vi "EnFlo_Hub.vi"() -> ()   [LabVIEW 2022 SP3]
uses:
  Anemometry Sub Vis/Controls/Launch_controls/Open_Calib.ctl
  Anemometry Sub Vis/Controls/Launch_controls/Open_Meas.ctl
  Anemometry Sub Vis/Controls/Launch_controls/Open_Enter_Temp.ctl
  Anemometry Sub Vis/Controls/Launch_controls/Multi_Run_Prog.ctl
  Anemometry Sub Vis/Controls/Launch_controls/EnFlo_arm.ctl
  Anemometry Sub Vis/Controls/Launch_controls/Disp_Setup.ctl
  Anemometry Sub Vis/Controls/Launch_controls/EnFlo_Tun_Setup.ctl
  Anemometry Sub Vis/Controls/Launch_controls/User_Metadata.ctl
  Anemometry Sub Vis/Controls/Launch_controls/Trav_3D_move.ctl
  Anemometry Sub Vis/Controls/Launch_controls/Trav_Space.ctl
  Anemometry Sub Vis/Controls/Launch_controls/Tunnel_speed.ctl
  Anemometry Sub Vis/Controls/Launch_controls/Client_source_control.ctl
  Anemometry Sub Vis/Controls/Launch_controls/Hydrosonic_Manual.ctl
  Anemometry Sub Vis/Controls/Launch_controls/Preference_Panel.ctl
  Anemometry Sub Vis/Controls/Launch_controls/Hot_wire_Calculator.ctl
  Anemometry Sub Vis/Controls/Launch_controls/RW_X_Parker_Config.ctl
  Anemometry Sub Vis/Controls/Launch_controls/LDA_Alignment.ctl
  Anemometry Sub Vis/Controls/Launch_controls/Named_Serial_Comms.ctl
  Anemometry Sub Vis/Controls/Launch_controls/BSA_data_rates.ctl
  Anemometry Sub Vis/Controls/Launch_controls/Serial_Setup.ctl
  Anemometry Sub Vis/Controls/Launch_controls/Post_Process_icon.ctl
  Anemometry Sub Vis/Controls/Launch_controls/Edit_Ascii_file.ctl
  Anemometry Sub Vis/Controls/Launch_controls/Edit_Raw_DF.ctl
  Anemometry Sub Vis/Controls/Launch_controls/Results_file_plotter.ctl
  Anemometry Sub Vis/Controls/Launch_controls/Serial_Port_Names.ctl
  Anemometry Sub Vis/Controls/Launch_controls/Paul.ctl
  Anemometry Sub Vis/Controls/Launch_controls/Tom.ctl
  Anemometry Sub Vis/Controls/Launch_controls/Scani_Valve.ctl
  Anemometry Sub Vis/Controls/Launch_controls/Edit_sever_Channel.ctl
  Anemometry Sub Vis/Controls/Launch_controls/Day_file_plotter.ctl
  Anemometry Sub Vis/Controls/Launch_controls/Plot_Sever_Data.ctl
  Anemometry Sub Vis/Controls/Launch_controls/Adam_Table.ctl
  Anemometry Sub Vis/Controls/Launch_controls/Active_Channel_Control.ctl
  Anemometry Sub Vis/Controls/Launch_controls/Laser on,off.ctl
  Anemometry Sub Vis/Controls/Launch_controls/Laser set power.ctl
  Anemometry Sub Vis/Controls/Preference_Mode.ctl
  Anemometry Sub Vis/Controls/Post_Process.ctl
  Anemometry Sub Vis/Controls/User_Specific_mode.ctl
  Anemometry Sub Vis/Controls/Serveds.ctl
  ADAM Client/Sub VIs/ADAM Controls/Ch_description_ADAM.ctl
  ADAM Client/Sub VIs/ADAM Controls/Module_type_ADAM.ctl
  ADAM Client/Sub VIs/ADAM Controls/Function_ADAM.ctl
  ADAM Client/Sub VIs/ADAM Controls/Channel_State.ctl
  ADAM Client/Sub VIs/ADAM Controls/Calib_type_ADAM.ctl
  ADAM Client/Sub VIs/ADAM Controls/Address.ctl
  Anemometry Sub Vis/Controls/Server_Comms.ctl
  ADAM Client/Sub VIs/ADAM Controls/Update_scan_value.ctl
  Anemometry Sub Vis/Controls/Setup.ctl
  Anemometry Sub Vis/Gen Trav/Trav_mode.ctl
  Anemometry Sub Vis/File/Setup_Filetype.ctl
  Anemometry Sub Vis/Calibration/Calib_mode.ctl
  Anemometry Sub Vis/Controls/App_Global.ctl
  239e5811-adcb-1c4c-a08f-5aaffcc560b3.vi
  2186acc1-5873-0847-b6a2-f2ea4a402273.vi
  Anemometry Sub Vis/Globals/Dynamic_call_global.ph.vi
  Anemometry Sub Vis/Globals/Meas_global.vi
  Anemometry Sub Vis/Utilities/Email_transfer_global.vi
  Anemometry Sub Vis/Globals/LDA_global.vi
  Anemometry Sub Vis/Globals/Preference_global.vi
  Anemometry Sub Vis/Globals/Constants_global.vi
  Camera Server/Globals/CamServer global.vi
  Anemometry Sub Vis/Globals/Trav_pos_global.vi
  Anemometry Sub Vis/Acquisition/PWA/PWAtasksGLOBAL.vi
  <vilib>/Platform/browser.llb/Open URL in Default Browser (string).vi
  <vilib>/Platform/browser.llb/Open URL in Default Browser (path).vi
  Anemometry Sub Vis/LDA/Coherent/Coherent global.vi
panel:
  out "PWA No. of Samples":i32=100
  in  "stop":bool
  out "CamServer machine name or IP":string="EnFlo-CamServer"
  out "List of ADAM channels to view":string[](array[string])
  out "List of ADAM control channels":string[](array[string])
  out "Numeric":i32
  out "Rig Name":string="EnFlo Tunnel"
  out "All Users":path=path "/System Folder/Preferences/LabVIEW (EnFlo specific)/Meas Setups"
  out "Dummy Measurement":bool
  in  "Tab Control":T1(tab)
  in  "Plot Meas Chs":bool
  in  "Mult Trav Move":bool
  in  "Tunnel Speed Control":T2
  in  "Traverse Space":T3
  in  "Trav 3D Move":T4 caption="3D Traverse Move"
  in  "User Metadata":T5
  in  "Multi Run Prog":T6
  in  "Enter Temp_Press":T7
  in  "Measurement Prog":T8 caption="Measurement"
  in  "Calibration Prog":T9 caption="Calibration"
  in  "LDA Control":bool
  in  "Beam Power Meter":bool
  in  "Source Live":bool
  in  "Laser set power":T10
  in  "Laser on/off":T11
  in  "Scani Valve":T12
  in  "LDA Alignment":T13
  in  "Hydrosonic Control":T14
  in  "Source Control":T15
  in  "Gas Release Setup":T16
  in  "EnFlo Tunnel Setup":T17
  in  "Heater Setup":bool caption="Inlet heater File"
  in  "EnFlo Arm":T18
  in  "EnFlo Tun Display":bool
  in  "Beam Check Positions":bool
  in  "Edit Channel Interactive":bool
  in  "Rig_Control":cluster{"Ch Name":string, "Boolean":bool}[](array[cluster])
  in  "ADAM Channels Control":T19 caption="Change Active Channels"
  in  "ADAM Scan Table":T20 caption="Run ADAM Scan Table"
  in  "Edit Server Channel":T21
  in  "Plot Server Channels":T22 caption="Plot Server Data"
  in  "Day Files Plotter":T23 caption="Plot Data From File"
  out "Current Values":cluster{"Ch Name":string, "Numeric":dbl}[](array[cluster])
  out "Tunnel Running?":bool
  in  "Post_Pro_Results_Hierarchy":bool
  in  "Results File Plotter":T24
  in  "Edit Raw Data Files":T25
  in  "Edit ASCII File":T26
  in  "Post Process Raw Data":T27
  in  "changelog":bool
  in  "HierarchyHealthcheck":bool
  in  "ResetFPs":bool
  in  "SaveFPs":bool
  in  "Move Mirror":bool
  in  "Display Bad Trav Points":bool
  in  "Plot_FFID_Calibs.vi":bool
  in  "Top Level Traverse":bool
  in  "Show Manual Sync":bool
  in  "Port Names":T28
  in  "Serial Setup":T29
  in  "LDA Data Rate":T30
  in  "Serial Comms":T31 caption="Named Serial Comms"
  in  "RW Trav Setup":T32
  in  "Hot Wire Calc":T33
  in  "Preference Panel":T34
  in  "Risk Assessments (Surrey)":bool
  out "Revision Info":string
  in  "Tom Lawton tlawton@cppwind.com":T35 caption="For -other- support"
  in  "Paul Hayden p.hayden@surrey.ac.uk":T36 caption="For software support"
  in  "Online Manual":bool
  out "VI Name":string
  out "Iterations":i32
  # "Or give us a call on Tel: 01483 689545"
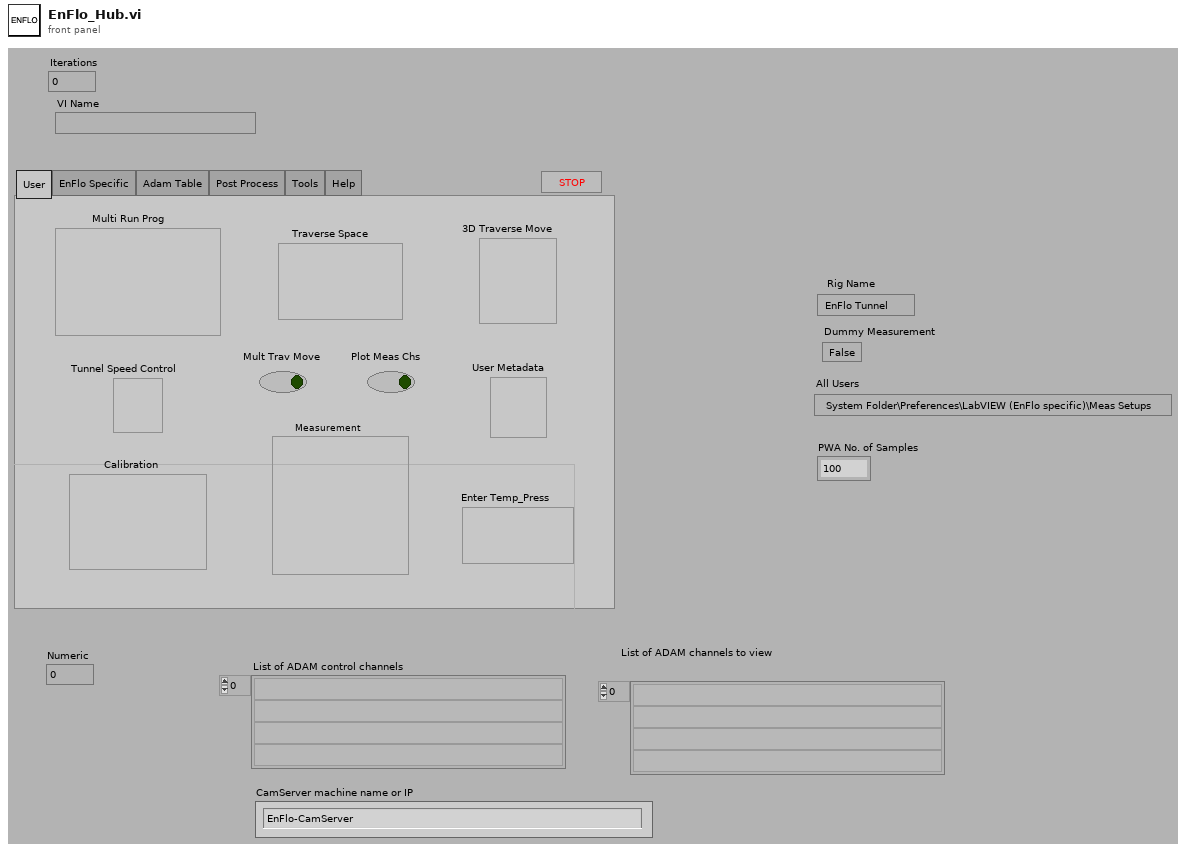
[diagram p1: front panel]
types:
  T1 = enum32{"User", "EnFlo Specific", "Adam Table", "Post Process", "Tools", "Help"}
  T2 = typedef "Tunnel_speed.ctl" = bool
  T3 = typedef "Trav_Space.ctl" = bool
  T4 = typedef "Trav_3D_move.ctl" = bool
  T5 = typedef "User_Metadata.ctl" = bool
  T6 = typedef "Multi_Run_Prog.ctl" = bool
  T7 = typedef "Open_Enter_Temp.ctl" = bool
  T8 = typedef "Open_Meas.ctl" = bool
  T9 = typedef "Open_Calib.ctl" = bool
  T10 = typedef "Laser set power.ctl" = bool
  T11 = typedef "Laser on,off.ctl" = bool
  T12 = typedef "Scani_Valve.ctl" = bool
  T13 = typedef "LDA_Alignment.ctl" = bool
  T14 = typedef "Hydrosonic_Manual.ctl" = bool
  T15 = typedef "Client_source_control.ctl" = bool
  T16 = typedef "Disp_Setup.ctl" = bool
  T17 = typedef "EnFlo_Tun_Setup.ctl" = bool
  T18 = typedef "EnFlo_arm.ctl" = bool
  T19 = typedef "Active_Channel_Control.ctl" = bool
  T20 = typedef "Adam_Table.ctl" = bool
  T21 = typedef "Edit_sever_Channel.ctl" = bool
  T22 = typedef "Plot_Sever_Data.ctl" = bool
  T23 = typedef "Day_file_plotter.ctl" = bool
  T24 = typedef "Results_file_plotter.ctl" = bool
  T25 = typedef "Edit_Raw_DF.ctl" = bool
  T26 = typedef "Edit_Ascii_file.ctl" = bool
  T27 = typedef "Post_Process_icon.ctl" = bool
  T28 = typedef "Serial_Port_Names.ctl" = bool
  T29 = typedef "Serial_Setup.ctl" = bool
  T30 = typedef "BSA_data_rates.ctl" = bool
  T31 = typedef "Named_Serial_Comms.ctl" = bool
  T32 = typedef "RW_X_Parker_Config.ctl" = bool
  T33 = typedef "Hot_wire_Calculator.ctl" = bool
  T34 = typedef "Preference_Panel.ctl" = bool
  T35 = typedef "Tom.ctl" = bool
  T36 = typedef "Paul.ctl" = bool
  T37 = typedef "Post_Process.ctl" = enum16{"Take New Data", "Post Process Raw Data File"}
  T38 = typedef "Preference_Mode.ctl" = enum16{"Load Preferences from file", "Save Preferences to file", "Load, Edit then Save"}
  T39 = typedef "User_Specific_mode.ctl" = enum16{"Check VI only", "Run VI"}
  T40 = typedef "Serveds.ctl" = enum16{"Read Global", "Load Global From File"}
  T41 = typedef "Server_Comms.ctl" = enum16{"Do Not Link To Server", "Server Link Healthy"}
  T42 = typedef "Ch_description_ADAM.ctl" = cluster{"Ch Name":string, "Type":T43, "Function":T44, "Ch State":T45, "Calibration type":T46, "A":dbl, "B":dbl, "C":dbl, "D":dbl, "Comments":string, "Address":T47, "String":string, "Duty":u16}
  T43 = typedef "Module_type_ADAM.ctl" = string
  T44 = typedef "Function_ADAM.ctl" = enum16{"Analogue Input", "Digital Input", "Event counter", "Event rate", "Analogue Output", "Digital Output", "Relay Output"}
  T45 = typedef "Channel_State.ctl" = enum16{"On", "Off", "Always On", "Always Off"}
  T46 = typedef "Calib_type_ADAM.ctl" = string
  T47 = typedef "Address.ctl" = cluster{"Main":i32, "Ch.":i32, "Sub":i32, "Port Name":string}
  T48 = typedef "Update_scan_value.ctl" = cluster{"Channel Name":string, "New Value":dbl, "!Auto_Off":bool}
  T49 = typedef "Setup.ctl" = enum16{"Run Program", "Show Setup", "Save Current Setup", "Setup Front Panel"}
  T50 = enum32{"Bad", "Idle", "Run top level", "Running"}
  T51 = enum16{"Get Channel Names", "Get Current Value", "Update Channel Value", "Update Channel Description"}
  T52 = enum32{"Invalid", "Standard", "Closed", "Hidden", "Minimized", "Maximized"}
  T53 = typedef "Trav_mode.ctl" = enum16{"Move traverse", "Read traverse position", "Teach Position"}
  T54 = typedef "Setup_Filetype.ctl" = enum16{"Measurement Setups", "Calibration Setups", "General", "Results File Plotter Setups", "Speed Calib Tweaks"}
  T55 = enum16{"Load Command File", "Save Command File", "Check Multi Run Prog", "Check Multi Run Prog With Live Moves", "Run Multi Run Prog"}
  T56 = typedef "Calib_mode.ctl" = enum16{"Show Setup", "Take a New Calibration Point", "Refit Curve", "Setup Front Panel"}
  T57 = typedef "App_Global.ctl" = enum16{"Read Global", "Write to Global", "Initialise Array"}
  T58 = cluster{"Shift":bool, "Ctrl":bool, "Alt":bool, "Cmd":bool, "Opt":bool}
  T59 = typedef "Tunnel_Coordinates.ctl" = enum16{"Work in Tunnel Coordinates", "Work in Model Coordinates"}
  T60 = typedef "App_Ref_Cluster.ctl" = cluster{"Server IP & Port No":string, "Application reference":refnum<vi>}
  T61 = typedef "Monitor values.ctl" = cluster{"Power (mW)":sgl, "LDD current (A)":sgl, "TEC drive (V)":sgl, "TEC temp. (degC)":sgl, "SHG heater (degC)":sgl, "BRF heater (degC)":sgl}
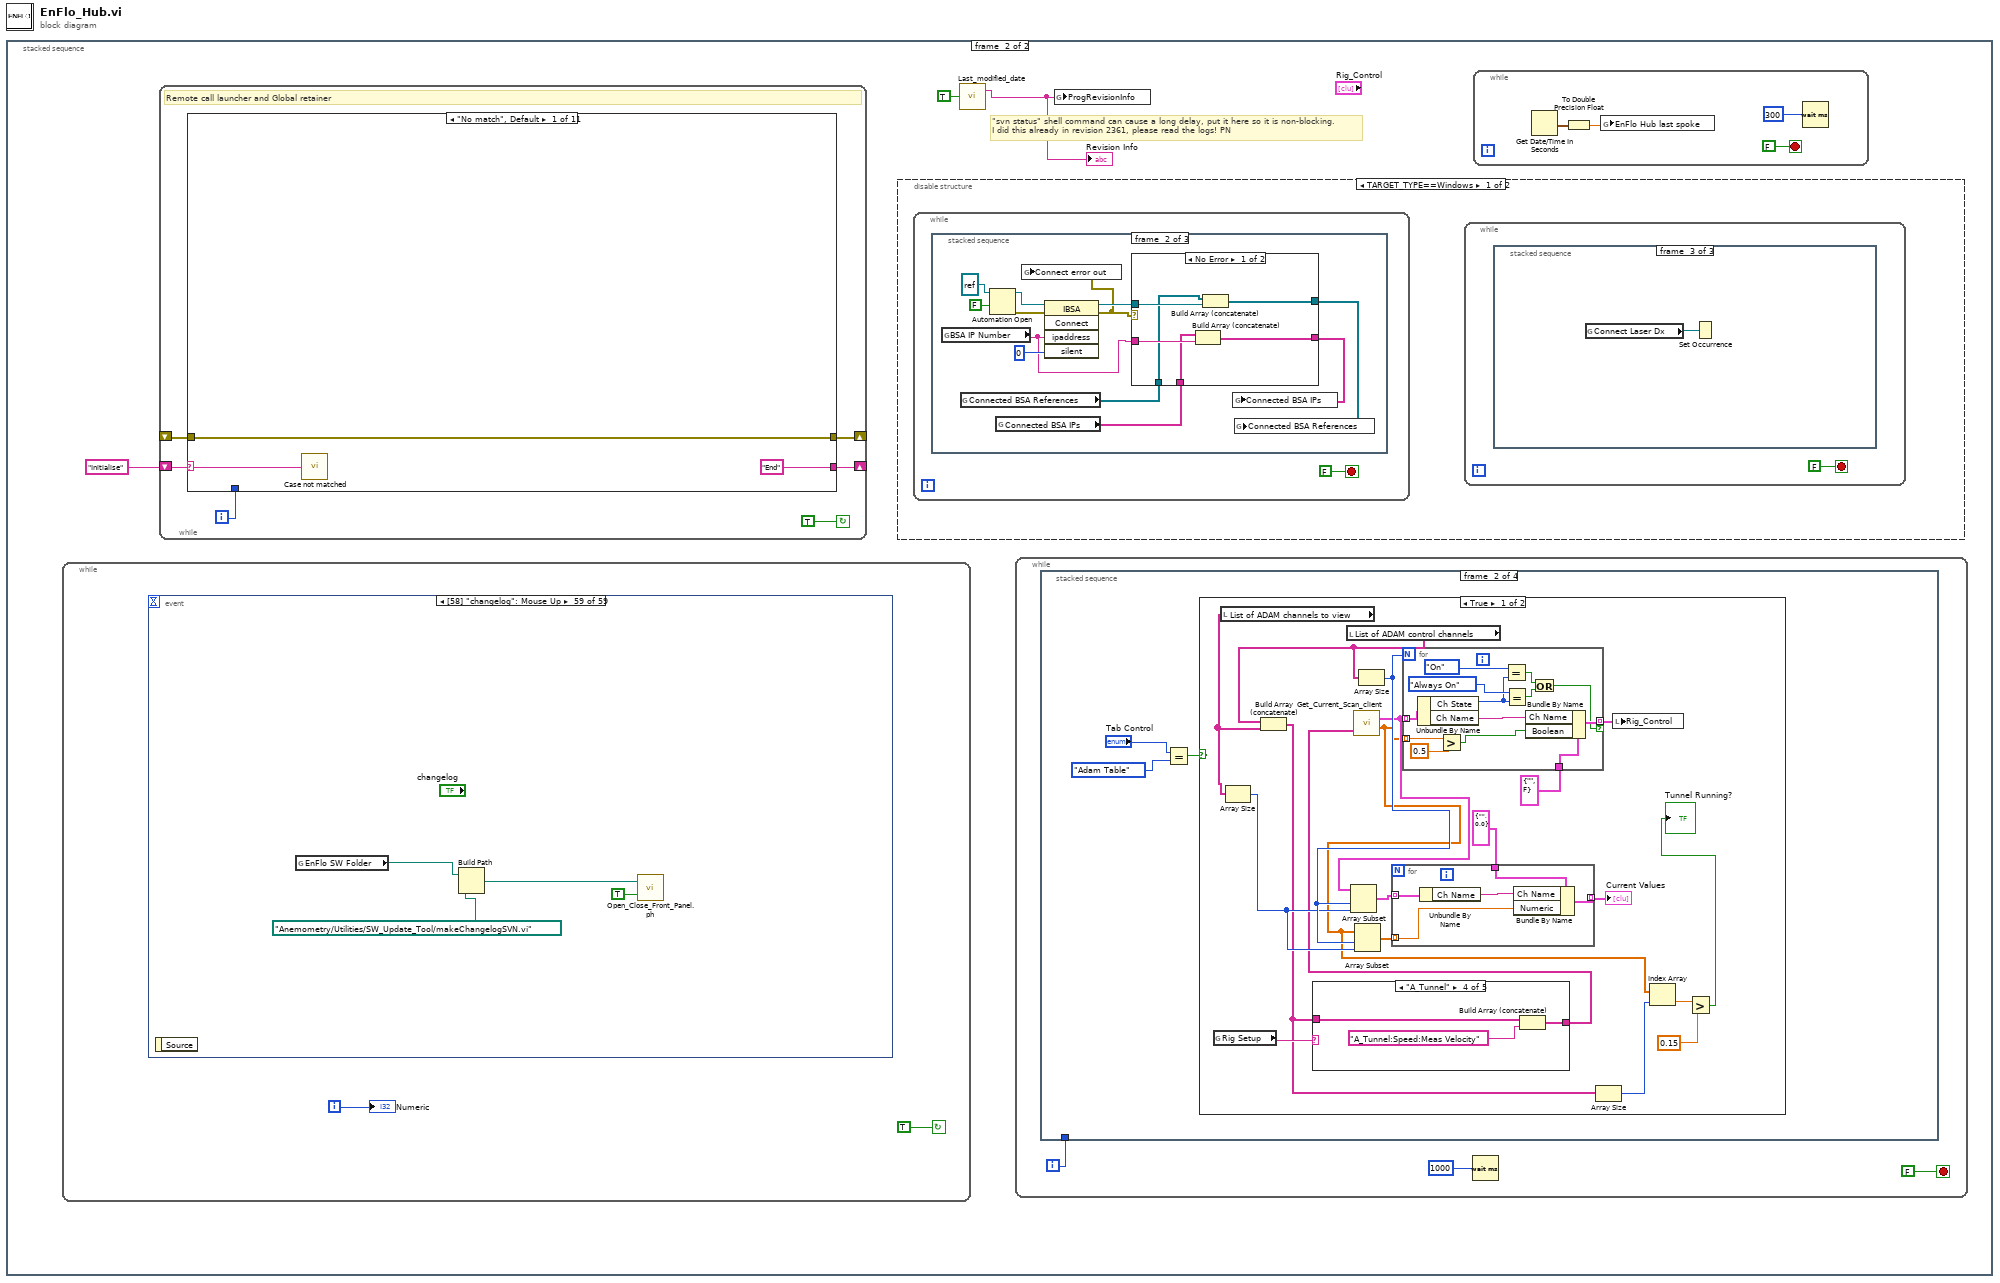
[diagram p0: block diagram]
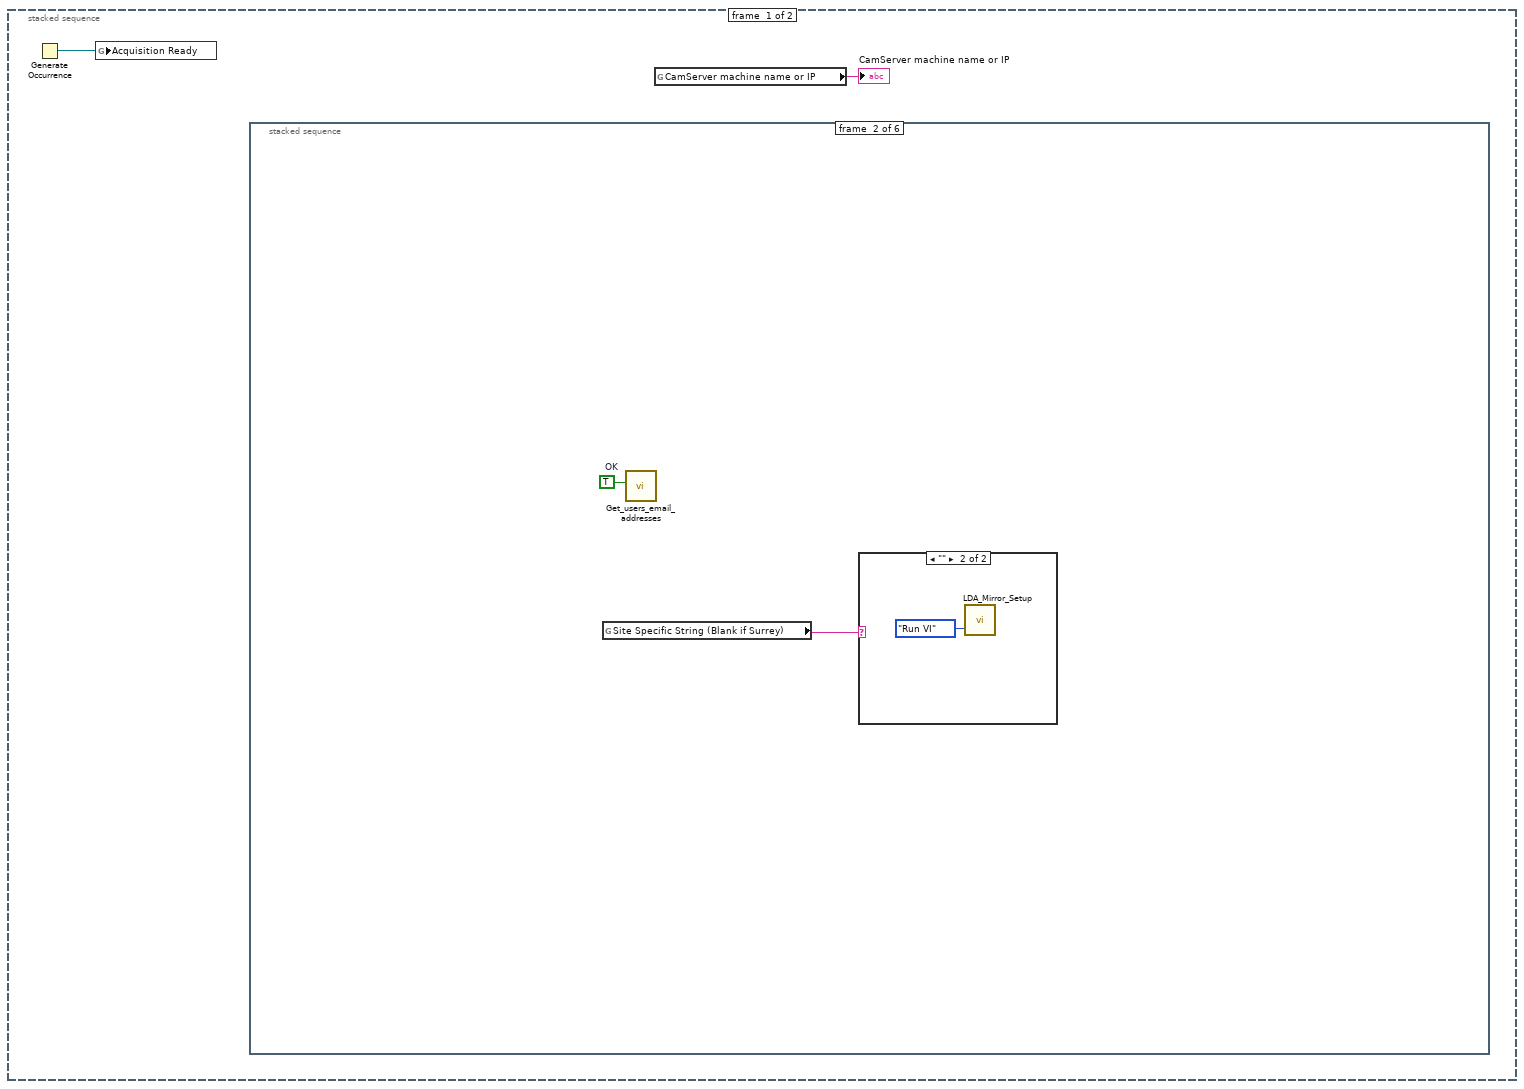
[diagram p2: hidden frame]
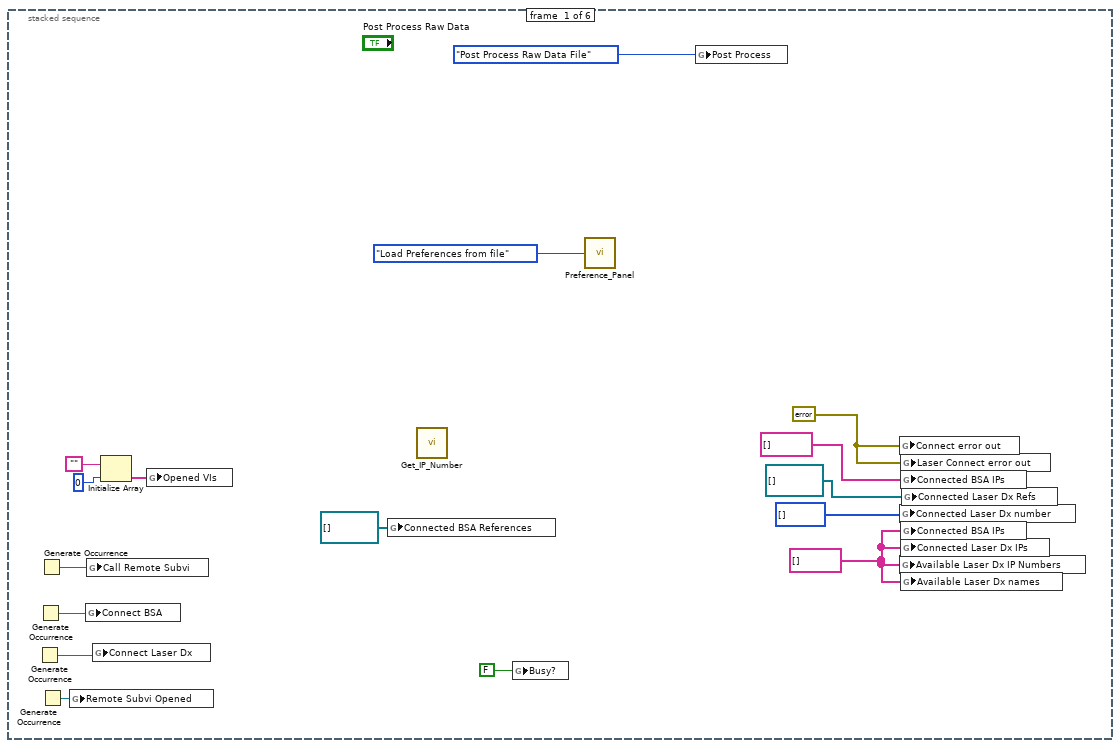
[diagram p3: hidden frame]
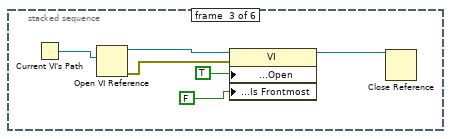
[diagram p5: hidden frame]
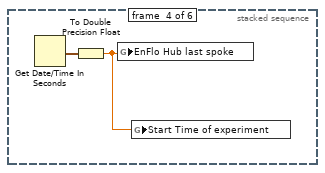
[diagram p6: hidden frame]
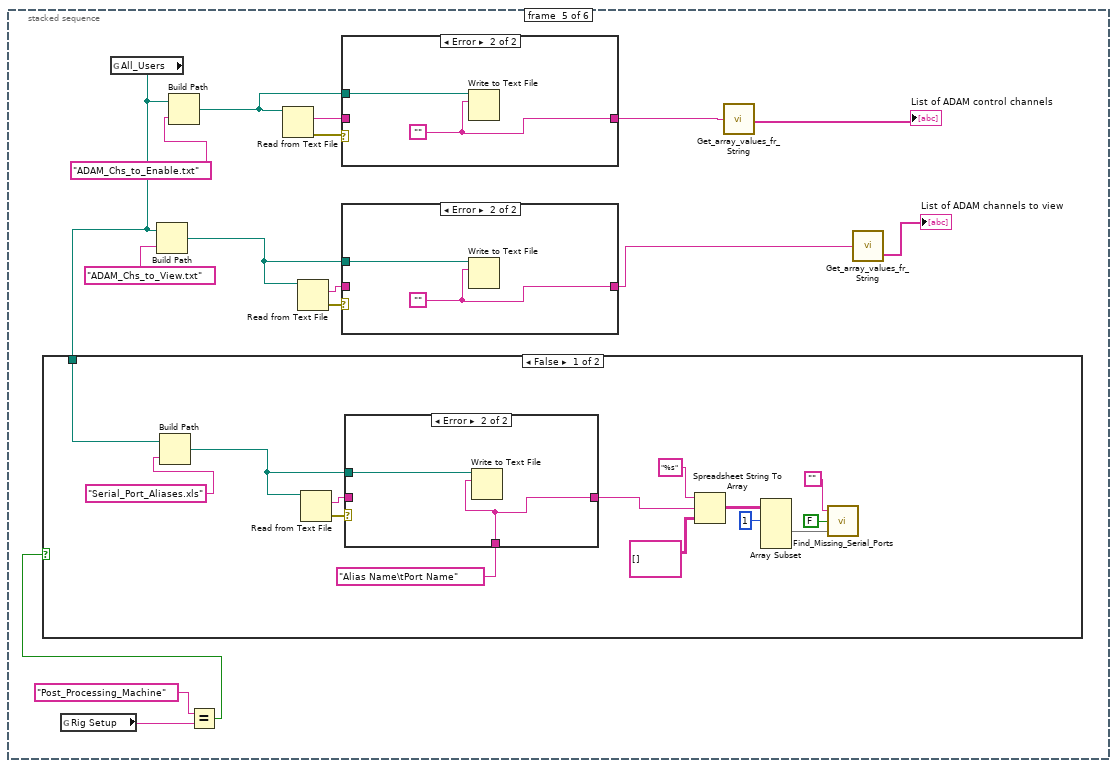
[diagram p7: hidden frame]
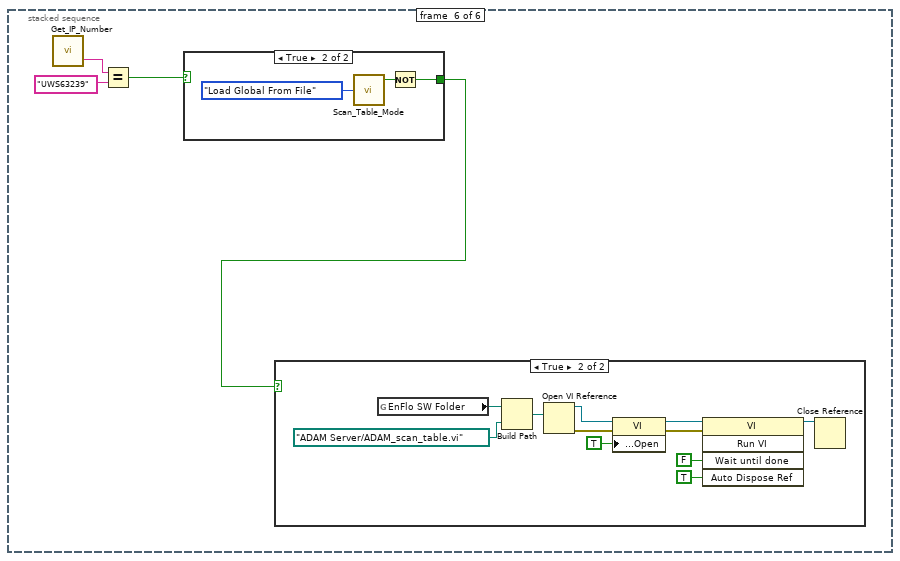
[diagram p12: hidden frame]
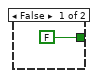
[diagram p14: hidden frame]
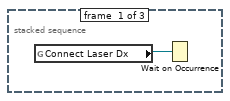
[diagram p15: hidden frame]
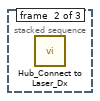
[diagram p16: hidden frame]
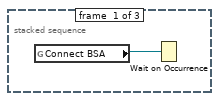
[diagram p17: hidden frame]
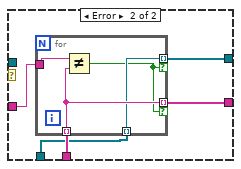
[diagram p18: hidden frame]
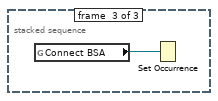
[diagram p19: hidden frame]
diagram:
  n1 = stacked-sequence {
    frame #0 {
      n2 = Generate Occurrence() -> (w2:refnum<k4>)
      n3 = global write "Meas_global.vi" "Acquisition Ready"(w2) -> ()
      n4 = stacked-sequence {
        frame #0 {
          w6 = errorcluster {"status"=FALSE, "code"=0, "source"=""} ("error out")
          w5 = string[] [] ("Connected Laser Dx IPs")
          n5 = Generate Occurrence() -> (w9:refnum<k4>)
          n6 = Generate Occurrence() -> (w11:refnum<k4>)
          n7 = Generate Occurrence() -> (w18:refnum<k4>)
          n8 = Generate Occurrence() -> (w17:refnum<k4>)
          n9 = global write "Dynamic_call_global.ph.vi" "Remote Subvi Opened"(w17) -> ()
          n10 = global write "LDA_global.vi" "Connect BSA"(w11) -> ()
          n11 = global write "Dynamic_call_global.ph.vi" "Call Remote Subvi"(w18) -> ()
          n12 = global write "LDA_global.vi" "Connect Laser Dx"(w9) -> ()
          n13 = Initialize Array("", 0) -> (w15:string[])
          n14 = global write "Dynamic_call_global.ph.vi" "Opened VIs"(w15) -> ()
          n15 = global write "LDA_global.vi" "Connected BSA References"(refnum<k7>[] [] ("Connected BSA References")) -> ()
          n16 = call "Get_IP_Number.vi"() -> ()  [unwired: 2 out]
          n17 = global write "Email_transfer_global.vi" "Busy?"(FALSE ("Busy?")) -> ()
          n18 = call "Preference_Panel.vi"("Mode"=Preference_Mode."Load Preferences from file") -> ()
          n19 = global write "Meas_global.vi" "Post Process"(Post_Process."Post Process Raw Data File" ("Post Process")) -> ()
          n20 = global write "LDA_global.vi" "Connect error out"(w6) -> ()
          n21 = global write "LDA_global.vi" "Connected Laser Dx number"(i64[] [] ("Connected Laser Dx number")) -> ()
          n22 = global write "LDA_global.vi" "Available Laser Dx IP Numbers"(w5) -> ()
          n23 = global write "LDA_global.vi" "Laser Connect error out"(w6) -> ()
          n24 = global write "LDA_global.vi" "Connected BSA IPs"(string[] []) -> ()
          n25 = global write "LDA_global.vi" "Connected BSA IPs"(w5) -> ()
          n26 = global write "LDA_global.vi" "Connected Laser Dx IPs"(w5) -> ()
          n27 = global write "LDA_global.vi" "Available Laser Dx names"(w5) -> ()
          n28 = global write "LDA_global.vi" "Connected Laser Dx Refs"(refnum<k7>[] [] ("Connected Laser Dx Refs")) -> ()
        }
        frame #1 {
          w20 = TRUE  # OK
          n29 = global read "Preference_global.vi" "Site Specific String (Blank if Surrey)"() -> (w19:string)
          n30 = call "Get_users_email_addresses.vi"("OK"=w20) -> ()  [unwired: 5 out]
          n31 = case shown="\"\"" w19 {
            frame "CPP", Default {
            }
            frame "" {
              n32 = call "LDA_Mirror_Setup.vi"("Simulate/Run"=User_Specific_mode."Run VI") -> ()  [unwired: 3 in, 1 out]
            }
          }
        }
        frame #2 {
          n33 = Current VI's Path() -> (path=w27:path)
          n34 = Open VI Reference(vi path=w27) -> (vi reference=w26:refnum<vi>, error out=w25:errorcluster)  [unwired: 1 in, 4 out]
          n35 = property class="VI"(reference=w26, error in=w25, "Front Panel Window:Open"=TRUE, "Front Panel Window:Is Frontmost"=FALSE) -> (reference out=w24:refnum<vi>)  [unwired: 1 out]
          n36 = Close Reference(reference=w24) -> ()  [unwired: 1 in, 1 out]
        }
        frame #3 {
          n37 = Get Date/Time In Seconds() -> (seconds since 1Jan1904=w29:timestamp)
          n38 = To Double Precision Float(number=w29) -> (double precision float=w28:dbl)
          n39 = global write "Dynamic_call_global.ph.vi" "EnFlo Hub last spoke"(w28) -> ()
          n40 = global write "Meas_global.vi" "Start Time of experiment"(w28) -> ()
        }
        frame #4 {
          n41 = global read "Preference_global.vi" "Rig Setup"() -> (w31:string)
          n42 = global read "Constants_global.vi" "All_Users"() -> (w33:path)
          n43 = Build Path(base path=w33, name or relative path="ADAM_Chs_to_View.txt") -> (appended path=w36:path)
          n44 = Build Path(base path=w33, name or relative path="ADAM_Chs_to_Enable.txt") -> (appended path=w38:path)
          n45 = Equal?(x="Post_Processing_Machine" ("Rig Setup"), y=w31) -> (x = y?=w30:bool)
          n46 = case shown="False" w30 {
            tunnel: w33 -> [w57 _]
            frame False {
              n47 = Build Path(base path=w57, name or relative path="Serial_Port_Aliases.xls") -> (appended path=w50:path)
              n48 = Read from Text File(file (use dialog)=w50) -> (text=w59:string, error out=w58:errorcluster)  [unwired: 3 in, 2 out]
              n49 = case shown="Error" w58 {
                tunnel: [w60 w61] -> w55
                tunnel: w59 -> [w60 _]
                tunnel: w50 -> [_ w62]
                tunnel: "Alias Name\tPort Name" -> [_ w61]
                frame No Error {
                }
                frame Error {
                  n50 = Write to Text File(file (use dialog)=w62, text=w61) -> ()  [unwired: 2 in, 3 out]
                }
              }
              n51 = Spreadsheet String To Array(format string="%s", spreadsheet string=w55, array type (2D Dbl)=string[][] []) -> (array=w53:string[][])  [unwired: 1 in]
              n52 = Array Subset(array=w53, index (row)=1 ("index")) -> (w49:string[][])  [unwired: 3 in]
              n53 = call "Find_Missing_Serial_Ports.vi"("Serial Port Aliases"=w49, "Must have Port?"=FALSE, "Aliase to Check"="") -> ()  [unwired: 1 out]
            }
            frame True {
            }
          }
          n54 = Read from Text File(file (use dialog)=w38) -> (text=w39:string, error out=w41:errorcluster)  [unwired: 3 in, 2 out]
          n55 = Read from Text File(file (use dialog)=w36) -> (text=w34:string, error out=w35:errorcluster)  [unwired: 3 in, 2 out]
          n56 = case shown="Error" w41 {
            tunnel: [w66 w68] -> w40
            tunnel: w39 -> [w66 _]
            tunnel: w38 -> [_ w67]
            frame No Error {
            }
            frame Error {
              w68 = ""
              n57 = Write to Text File(file (use dialog)=w67, text=w68) -> ()  [unwired: 2 in, 3 out]
            }
          }
          n58 = case shown="Error" w35 {
            tunnel: [w63 w65] -> w37
            tunnel: w34 -> [w63 _]
            tunnel: w36 -> [_ w64]
            frame No Error {
            }
            frame Error {
              w65 = ""
              n59 = Write to Text File(file (use dialog)=w64, text=w65) -> ()  [unwired: 2 in, 3 out]
            }
          }
          n60 = call "Get_array_values_fr_String.vi"("String Value"=w40) -> ("String array"=→"List of ADAM control channels":string[])  [unwired: 1 out]
          n61 = call "Get_array_values_fr_String.vi"("String Value"=w37) -> ("String array"=→"List of ADAM channels to view":string[])  [unwired: 1 out]
        }
        frame #5 {
          n62 = call "Get_IP_Number.vi"() -> ("bestAvailableName"=w71:string)  [unwired: 1 out]
          n63 = Equal?(x=w71, y="UWS63239" ("Computer Name")) -> (x = y?=w70:bool)
          n64 = case shown="True" w70 {
            tunnel: [FALSE w85] -> w69
            frame False {
            }
            frame True {
              n65 = call "Scan_Table_Mode.vi"("Mode"=Serveds."Load Global From File") -> ("Simulate Mode ?"=w86:bool)  [unwired: 2 out]
              n66 = Not(x=w86) -> (.not. x?=w85:bool)
            }
          }
          n67 = case shown="True" w69 {
            frame False {
            }
            frame True {
              n68 = global read "Constants_global.vi" "EnFlo SW Folder"() -> (w81:path)
              n69 = Build Path(base path=w81, name or relative path=path "ADAM Server/ADAM_scan_table.vi") -> (appended path=w82:path)
              n70 = Open VI Reference(vi path=w82) -> (vi reference=w79:refnum<vi>, error out=w78:errorcluster)  [unwired: 1 in, 4 out]
              n71 = property class="VI"(reference=w79, error in=w78, "Front Panel Window:Open"=TRUE) -> (reference out=w76:refnum<vi>, error out=w75:errorcluster)
              n72 = invoke class="VI" method="Run VI"(reference=w76, error in=w75, "Wait until done"=FALSE, "Auto Dispose Ref"=TRUE) -> (reference out=w83:refnum<vi>)  [unwired: 1 in, 4 out]
              n73 = Close Reference(reference=w83) -> ()  [unwired: 1 in, 1 out]
            }
          }
        }
      }
      n74 = global read "CamServer global.vi" "CamServer machine name or IP"() -> (→"CamServer machine name or IP":string)
    }
    frame #1 {
      # "\"svn status\" shell command can cause a long delay, put it here so it is non-blocking.\nI did this already in revision 2361, please read the logs! PN"
      n75 = while {
        i -> [w386]
        stop <- TRUE continue-if-true
        n76 = event shown="[58] \"changelog\": Mouse Up" {
          selector: _ -> [_ _ _ _ _ _ _ _ _ _ _ _ _ _ _ _ _ _ _ _ _ _ _ _ _ _ _ _ _ _ _ _ _ _ _ _ _ _ _ _ _ _ _ _ _ _ _ _ _ _ _ _ _ _ _ _ _ _ _]
          dyn-events: _ -> [_ _ _ _ _ _ _ _ _ _ _ _ _ _ _ _ _ _ _ _ _ _ _ _ _ _ _ _ _ _ _ _ _ _ _ _ _ _ _ _ _ _ _ _ _ _ _ _ _ _ _ _ _ _ _ _ _ _ _]
          timeout: _ -> [_ _ _ _ _ _ _ _ _ _ _ _ _ _ _ _ _ _ _ _ _ _ _ _ _ _ _ _ _ _ _ _ _ _ _ _ _ _ _ _ _ _ _ _ _ _ _ _ _ _ _ _ _ _ _ _ _ _ _]
          event Mouse Down? {
            w396 = "Measurement.vi" ("name or relative path")
            n77 = event-data() -> ()  [unwired: 2 out]
            n78 = global read "Constants_global.vi" "EnFlo SW Folder"() -> (w399:path)
            n79 = Open VI Reference(vi path=w396) -> (vi reference=w395:refnum<vi>, error out=w394:errorcluster)  [unwired: 1 in, 4 out]
            n80 = Build Path(base path=w399, name or relative path="Anemometry") -> (appended path=w402:path)
            n81 = property class="VI"(reference=w395, error in=w394, "Front Panel Window:Open"=TRUE) -> (reference out=w393:refnum<vi>, error out=w388:errorcluster)
            n82 = Build Path(base path=w402, name or relative path=w396) -> (appended path=w400:path)
            n83 = global read "Preference_global.vi" "Rig Setup"() -> (w391:string)
            n84 = Close Reference(reference=w393, error in (no error)=w388) -> (error out=w392:errorcluster)
            n85 = Unbundle By Name(w392) -> ("status"=w401:bool)
            n86 = Equal?(x="Post_Processing_Machine" ("Rig Setup"), y=w391) -> (x = y?=w389:bool)
            n87 = case shown="True" w401 {
              tunnel: w400 -> [_ w405]
              tunnel: w392 -> [_ _]
              tunnel: w389 -> [_ w404]
              frame False {
              }
              frame True {
                n88 = stacked-sequence {
                  tunnel: w405 -> [w414 _]
                  tunnel: w404 -> [w406 _]
                  frame #0 {
                    n89 = Open VI Reference(type specifier VI Refnum (for type only)=refnum<vi> refnum, vi path=w414) -> (vi reference=w412:refnum<vi>, error out=w411:errorcluster)  [unwired: 1 in, 3 out]
                    n90 = property class="VI Interface Type 4"(reference=w412, error in=w411, "Front Panel Window:Open"=TRUE) -> (reference out=w408:refnum<vi>, error out=w407:errorcluster)
                    n91 = case shown="False" w406 {
                      tunnel: [w420 w422] -> w410
                      tunnel: [w419 w421] -> _
                      tunnel: w408 -> [w418 w422]
                      tunnel: w407 -> [w417 w421]
                      frame False {
                        n92 = call-by-ref "?"(reference=w418, error in=w417, "setup"=Setup."Setup Front Panel", "Post Process"=Post_Process."Take New Data") -> (reference out=w420:refnum<vi>, error out=w419:errorcluster)  [unwired: 16 in, 2 out]
                      }
                      frame True {
                      }
                    }
                    n93 = Close Reference(reference=w410) -> ()  [unwired: 1 in, 1 out]
                  }
                  frame #1 {
                    n94 = global write "Meas_global.vi" "Post Process"(Post_Process."Post Process Raw Data File" ("Post Process")) -> ()
                  }
                }
              }
            }
            n95 = event-data("Discard?"=TRUE) -> ()  [unwired: 1 in, 2 out]
          }
          event Mouse Down? {
            n96 = event-data() -> ()  [unwired: 2 out]
            n97 = call-poly <vilib>:"Open URL in Default Browser.vi"("URL"="Mailto:tlawton@cppwind.com") -> ()  [unwired: 1 in, 6 out]
            n98 = event-data() -> ()  [unwired: 1 in, 5 out]
          }
          event Mouse Down? {
            n99 = event-data() -> ()  [unwired: 5 out]
            n100 = call-poly <vilib>:"Open URL in Default Browser.vi"("URL"="Mailto:p.hayden@surrey.ac.uk") -> ()  [unwired: 1 in, 6 out]
            n101 = event-data() -> ()  [unwired: 1 in, 2 out]
          }
          event "Online Manual": Mouse Down? {
            n102 = event-data() -> ()  [unwired: 2 out]
            n103 = global read "Constants_global.vi" "EnFlo SW Folder"() -> (w428:path)
            n104 = Build Path(base path=w428, name or relative path="Manuals\\online\\index.html" ("URL")) -> (appended path=w426:path)
            n105 = call-poly <vilib>:"Open URL in Default Browser.vi"("path"=w426) -> ()  [unwired: 1 in, 6 out]
            n106 = event-data() -> ()  [unwired: 1 in, 2 out]
          }
          event "Risk Assessments (Surrey)": Mouse Down? {
            n107 = event-data() -> ()  [unwired: 9 out]
            n108 = global read "Constants_global.vi" "EnFlo SW Folder"() -> (w432:path)
            n109 = Build Path(base path=w432, name or relative path=path "Manuals/online/Surrey_Risk_Assessments _URL.txt") -> (appended path=w430:path)
            n110 = Read from Text File(file (use dialog)=w430) -> (text=w429:string)  [unwired: 3 in, 3 out]
            n111 = call <vilib>:"Open URL in Default Browser core.vi"("url"=w429) -> ()  [unwired: 5 in, 2 out]
            n112 = event-data() -> ()  [unwired: 5 in, 1 out]
          }
          event Mouse Down? {
            n113 = event-data() -> ()  [unwired: 9 out]
            n114 = global read "Constants_global.vi" "EnFlo SW Folder"() -> (w433:path)
            n115 = Build Path(base path=w433, name or relative path=path "ADAM Client/ADAM client VIs/ScaniValve_client.vi") -> (appended path=w436:path)
            n116 = call "Open_Close_Front_Panel.ph.vi"("openWindow (T)"=TRUE ("Front Panel Window:Open"), "VI path"=w436) -> ()  [unwired: 1 in, 1 out]
            n117 = event-data() -> ()  [unwired: 1 in, 5 out]
          }
          event Mouse Down? {
            n118 = event-data() -> ()  [unwired: 9 out]
            n119 = global read "Constants_global.vi" "EnFlo SW Folder"() -> (w437:path)
            n120 = Build Path(base path=w437, name or relative path=path "Anemometry/Anemometry Sub Vis/LDA/Coherent/Laser power on,off (simple).vi") -> (appended path=w440:path)
            n121 = call "Open_Close_Front_Panel.ph.vi"("openWindow (T)"=TRUE ("Front Panel Window:Open"), "VI path"=w440) -> ()  [unwired: 1 in, 1 out]
            n122 = event-data() -> ()  [unwired: 2 in, 1 out]
          }
          event "LDA Control": Mouse Down? {
            n123 = event-data() -> ()  [unwired: 9 out]
            n124 = global read "Constants_global.vi" "EnFlo SW Folder"() -> (w450:path)
            n125 = Build Path(base path=w450, name or relative path=path "Anemometry/Anemometry Sub Vis/LDA/LDA Control.vi") -> (appended path=w441:path)
            n126 = Open VI Reference(vi path=w441) -> (vi reference=w445:refnum<vi>, error out=w447:errorcluster)  [unwired: 1 in, 4 out]
            n127 = property class="VI"(reference=w445, error in=w447, "Front Panel Window:Open"=TRUE) -> (reference out=w449:refnum<vi>, error out=w448:errorcluster)
            n128 = invoke class="VI" method="Run VI"(reference=w449, error in=w448, "Wait until done"=FALSE, "Auto Dispose Ref"=TRUE) -> (reference out=w442:refnum<vi>)  [unwired: 1 in, 4 out]
            n129 = Close Reference(reference=w442) -> ()  [unwired: 1 in, 1 out]
            n130 = event-data() -> ()  [unwired: 5 in, 1 out]
          }
          event "Source Live": Value Change {
            n131 = event-data() -> ()  [unwired: 7 out]
            n132 = flat-sequence {
              frame #0 {
                n133 = global read "Constants_global.vi" "EnFlo SW Folder"() -> (w452:path)
                n134 = Build Path(base path=w452, name or relative path=path "ADAM Serial/Instrument drivers/Arduino/Source_Live_Control_Manual.vi") -> (appended path=w455:path)
                n135 = call "Open_Close_Front_Panel.ph.vi"("openWindow (T)"=TRUE ("Front Panel Window:Open"), "VI path"=w455) -> ()  [unwired: 1 in, 1 out]
              }
              frame #1 {
                n136 = local write "Source Live"(FALSE) -> ()
              }
            }
          }
          event Mouse Down? {
            n137 = event-data() -> ()  [unwired: 9 out]
            n138 = global read "Constants_global.vi" "EnFlo SW Folder"() -> (w457:path)
            n139 = Build Path(base path=w457, name or relative path=path "Anemometry/Anemometry Sub Vis/LDA/Coherent/Set lasers power.vi") -> (appended path=w460:path)
            n140 = call "Open_Close_Front_Panel.ph.vi"("openWindow (T)"=TRUE ("Front Panel Window:Open"), "VI path"=w460) -> ()  [unwired: 1 in, 1 out]
            n141 = event-data() -> ()  [unwired: 2 in, 1 out]
          }
          event Mouse Down? {
            n142 = event-data() -> ()  [unwired: 5 out]
            n143 = global read "Constants_global.vi" "EnFlo SW Folder"() -> (w461:path)
            n144 = Build Path(base path=w461, name or relative path=path "ADAM Client/ADAM client VIs/Day_File_Plotter.vi") -> (appended path=w466:path)
            n145 = Open VI Reference(vi path=w466) -> (vi reference=w467:refnum<vi>, error out=w469:errorcluster)  [unwired: 2 in, 3 out]
            n146 = property class="VI"(reference=w467, error in=w469, "Front Panel Window:Open"=TRUE) -> (reference out=w471:refnum<vi>, error out=w470:errorcluster)
            n147 = invoke class="VI" method="Run VI"(reference=w471, error in=w470, "Wait until done"=FALSE, "Auto Dispose Ref"=TRUE) -> (reference out=w463:refnum<vi>)  [unwired: 1 in, 4 out]
            n148 = Close Reference(reference=w463) -> ()  [unwired: 1 in, 1 out]
            n149 = event-data() -> ()  [unwired: 1 in, 4 out]
          }
          event Mouse Down? {
            n150 = event-data() -> ()  [unwired: 5 out]
            n151 = global read "Constants_global.vi" "EnFlo SW Folder"() -> (w472:path)
            n152 = Build Path(base path=w472, name or relative path=path "ADAM Serial/Serial Link Layer/subVIs/Port_Names.vi") -> (appended path=w474:path)
            n153 = Open VI Reference(vi path=w474) -> (vi reference=w478:refnum<vi>, error out=w479:errorcluster)  [unwired: 1 in, 4 out]
            n154 = invoke class="VI" method="Run VI"(reference=w478, error in=w479, "Wait until done"=TRUE, "Auto Dispose Ref"=TRUE) -> (reference out=w475:refnum<vi>)  [unwired: 1 in, 4 out]
            n155 = Close Reference(reference=w475) -> ()  [unwired: 1 in, 1 out]
            n156 = event-data() -> ()  [unwired: 1 in, 5 out]
          }
          event Mouse Up {
            # "Don't check for errors, so FP will always open even if button push fails"
            # "Shift-click to press \"flush\" button, if RFP not already running"
            n157 = event-data() -> ("PlatMods"=w502:T58)  [unwired: 8 out]
            n158 = global read "Constants_global.vi" "EnFlo SW Folder"() -> (w503:path)
            n159 = Build Path(base path=w503, name or relative path=path "Data plotting/Results_file_Plotter.vi") -> (appended path=w501:path)
            n160 = Unbundle By Name(w502) -> ("Ctrl"=w490:bool, "Shift"=w482:bool, "Alt"=w485:bool, "Opt"=w480:bool)
            n161 = Open VI Reference(vi path=w501) -> (vi reference=w492:refnum<vi>, error out=w495:errorcluster)  [unwired: 1 in, 4 out]
            n162 = property class="VI"(reference=w492) -> ("Exec.State"=w489:T50)  [unwired: 1 in, 2 out]
            n163 = Compound Arithmetic op=OR(w482, w485, w480) -> (w486:bool)
            n164 = Equal?(x=w489, y=T50."Idle" ("Execution:State")) -> (x = y?=w487:bool)
            n165 = And(x=w486, y=w487) -> (x .and. y?=w491:bool)
            n166 = Select(t="flushAll" ("Control Name"), s=w482, f="loadSetup") -> (s? t:f=w481:string)
            n167 = case shown="True" w491 {
              tunnel: w492 -> [w514 w519]
              tunnel: w495 -> [w513 w516]
              tunnel: [w514 w518] -> w494
              tunnel: [w513 w516] -> w493
              tunnel: w481 -> [_ w515]
              frame False {
              }
              frame True {
                n168 = invoke class="VI" method="Ctrl Val.Set"(reference=w519, "Control Name"=w515, "Value"=TRUE) -> (reference out=w518:refnum<vi>)  [unwired: 2 in, 4 out]
              }
            }
            n169 = property class="VI"(reference=w494, error in=w493, "Front Panel Window:Open"=TRUE) -> (reference out=w499:refnum<vi>, error out=w500:errorcluster)
            n170 = case shown="False" w490 {
              tunnel: w500 -> [w508 w511]
              tunnel: w499 -> [w507 w512]
              tunnel: [w506 w512] -> w497
              tunnel: [w505 w511] -> w496
              frame False {
                n171 = invoke class="VI" method="Run VI"(reference=w507, error in=w508, "Wait until done"=FALSE, "Auto Dispose Ref"=TRUE) -> (reference out=w506:refnum<vi>, error out=w505:errorcluster)  [unwired: 1 in, 3 out]
              }
              frame True {
              }
            }
            n172 = Close Reference(reference=w497, error in (no error)=w496) -> ()  [unwired: 1 out]
          }
          event Mouse Down? {
            n173 = event-data() -> ()  [unwired: 5 out]
            n174 = global read "Constants_global.vi" "EnFlo SW Folder"() -> (w520:path)
            n175 = Build Path(base path=w520, name or relative path=path "Anemometry/Utilities/Post_Process_Raw_data.vi") -> (appended path=w522:path)
            n176 = call "Open_Close_Front_Panel.ph.vi"("openWindow (T)"=TRUE ("Front Panel Window:Open"), "VI path"=w522) -> ()  [unwired: 1 in, 1 out]
            n177 = event-data() -> ()  [unwired: 1 in, 5 out]
          }
          event Mouse Down? {
            n178 = event-data() -> ()  [unwired: 5 out]
            n179 = global read "Constants_global.vi" "EnFlo SW Folder"() -> (w524:path)
            n180 = Build Path(base path=w524, name or relative path=path "Anemometry/Anemometry Sub Vis/Data_plotting_vis/Edit_Raw_DF_Header.vi") -> (appended path=w526:path)
            n181 = call "Open_Close_Front_Panel.ph.vi"("openWindow (T)"=TRUE ("Front Panel Window:Open"), "VI path"=w526) -> ()  [unwired: 1 in, 1 out]
            n182 = event-data() -> ()  [unwired: 1 in, 5 out]
          }
          event Mouse Down? {
            n183 = event-data() -> ()  [unwired: 5 out]
            n184 = global read "Constants_global.vi" "EnFlo SW Folder"() -> (w528:path)
            n185 = Build Path(base path=w528, name or relative path=path "ADAM Serial/Serial Link Layer/subVIs/Serial_Setup.vi") -> (appended path=w530:path)
            n186 = Open VI Reference(vi path=w530) -> (vi reference=w534:refnum<vi>, error out=w535:errorcluster)  [unwired: 1 in, 4 out]
            n187 = invoke class="VI" method="Run VI"(reference=w534, error in=w535, "Wait until done"=TRUE, "Auto Dispose Ref"=TRUE) -> (reference out=w531:refnum<vi>)  [unwired: 1 in, 4 out]
            n188 = Close Reference(reference=w531) -> ()  [unwired: 1 in, 1 out]
            n189 = event-data() -> ()  [unwired: 1 in, 2 out]
          }
          event Mouse Down? {
            n190 = event-data() -> ()  [unwired: 5 out]
            n191 = global read "Constants_global.vi" "EnFlo SW Folder"() -> (w537:path)
            n192 = Build Path(base path=w537, name or relative path=path "ADAM Serial/Serial Link Layer/Named_Serial_Comms.vi") -> (appended path=w539:path)
            n193 = call "Open_Close_Front_Panel.ph.vi"("openWindow (T)"=TRUE ("Front Panel Window:Open"), "VI path"=w539) -> ()  [unwired: 1 in, 1 out]
            n194 = event-data() -> ()  [unwired: 1 in, 5 out]
          }
          event Mouse Down? {
            n195 = event-data() -> ()  [unwired: 5 out]
            n196 = global read "Constants_global.vi" "EnFlo SW Folder"() -> (w540:path)
            n197 = Build Path(base path=w540, name or relative path=path "Anemometry/Anemometry Sub Vis/LDA/LDA_data_rate.vi") -> (appended path=w542:path)
            n198 = call "Open_Close_Front_Panel.ph.vi"("openWindow (T)"=TRUE ("Front Panel Window:Open"), "VI path"=w542) -> ()  [unwired: 1 in, 1 out]
            n199 = event-data() -> ()  [unwired: 1 in, 2 out]
          }
          event Mouse Down? {
            n200 = event-data() -> ()  [unwired: 5 out]
            n201 = global read "Constants_global.vi" "EnFlo SW Folder"() -> (w553:path)
            n202 = Build Path(base path=w553, name or relative path=path "ADAM Client/ADAM client VIs/Control_Channel_Status.vi") -> (appended path=w544:path)
            n203 = Open VI Reference(vi path=w544) -> (vi reference=w547:refnum<vi>, error out=w545:errorcluster)  [unwired: 1 in, 4 out]
            n204 = property class="VI"(reference=w547, error in=w545, "Front Panel Window:Open"=TRUE) -> (reference out=w548:refnum<vi>, error out=w549:errorcluster)
            n205 = invoke class="VI" method="Run VI"(reference=w548, error in=w549, "Wait until done"=FALSE, "Auto Dispose Ref"=TRUE) -> (reference out=w550:refnum<vi>)  [unwired: 1 in, 4 out]
            n206 = Close Reference(reference=w550) -> ()  [unwired: 1 in, 1 out]
            n207 = event-data() -> ()  [unwired: 1 in, 2 out]
          }
          event Mouse Down? {
            n208 = event-data() -> ()  [unwired: 5 out]
            n209 = global read "Constants_global.vi" "EnFlo SW Folder"() -> (w555:path)
            n210 = Build Path(base path=w555, name or relative path=path "Anemometry/Utilities/LDA_Beam_Alignment.vi") -> (appended path=w557:path)
            n211 = call "Open_Close_Front_Panel.ph.vi"("openWindow (T)"=TRUE ("Front Panel Window:Open"), "VI path"=w557) -> ()  [unwired: 1 in, 1 out]
            n212 = event-data() -> ()  [unwired: 1 in, 5 out]
          }
          event Mouse Down? {
            w560 = FALSE  # Wait until done
            n213 = event-data() -> ()  [unwired: 5 out]
            n214 = call "Run_Enter_Temp.vi"("Wait until done"=w560) -> ()  [unwired: 1 out]
            n215 = event-data("Discard?"=TRUE) -> ()  [unwired: 1 in, 4 out]
          }
          event Mouse Down? {
            n216 = event-data() -> ()  [unwired: 5 out]
            n217 = global read "Constants_global.vi" "EnFlo SW Folder"() -> (w561:path)
            n218 = Build Path(base path=w561, name or relative path=path "Anemometry/Utilities/Edit_ASCI_file.vi") -> (appended path=w564:path)
            n219 = call "Open_Close_Front_Panel.ph.vi"("openWindow (T)"=TRUE ("Front Panel Window:Open"), "VI path"=w564) -> ()  [unwired: 1 in, 1 out]
            n220 = event-data() -> ()  [unwired: 1 in, 5 out]
          }
          event "Heater Setup": Mouse Down? {
            n221 = event-data() -> ()  [unwired: 5 out]
            n222 = global read "Constants_global.vi" "EnFlo SW Folder"() -> (w565:path)
            n223 = Build Path(base path=w565, name or relative path=path "Anemometry/Utilities/Create_Heater_Setpoints_File.vi") -> (appended path=w568:path)
            n224 = call "Open_Close_Front_Panel.ph.vi"("openWindow (T)"=TRUE ("Front Panel Window:Open"), "VI path"=w568) -> ()  [unwired: 1 in, 1 out]
            n225 = event-data() -> ()  [unwired: 1 in, 5 out]
          }
          event Mouse Down? {
            n226 = event-data() -> ()  [unwired: 5 out]
            n227 = global read "Constants_global.vi" "EnFlo SW Folder"() -> (w569:path)
            n228 = Build Path(base path=w569, name or relative path=path "ADAM Client/Sub VIs/Gas_Release_Control.vi") -> (appended path=w572:path)
            n229 = call "Open_Close_Front_Panel.ph.vi"("openWindow (T)"=TRUE ("Front Panel Window:Open"), "VI path"=w572) -> ()  [unwired: 1 in, 1 out]
            n230 = event-data() -> ()  [unwired: 1 in, 5 out]
          }
          event Mouse Down? {
            n231 = event-data() -> ()  [unwired: 5 out]
            n232 = global read "Constants_global.vi" "EnFlo SW Folder"() -> (w573:path)
            n233 = Build Path(base path=w573, name or relative path=path "ADAM Client/ADAM client VIs/Edit_Server_Channel.vi") -> (appended path=w582:path)
            n234 = Open VI Reference(type specifier VI Refnum (for type only)=refnum<vi> refnum, vi path=w582) -> (vi reference=w576:refnum<vi>, error out=w577:errorcluster)  [unwired: 1 in, 3 out]
            n235 = property class="VI Interface Type 5"(reference=w576, error in=w577, "Front Panel Window:Open"=TRUE) -> (reference out=w579:refnum<vi>, error out=w580:errorcluster)
            n236 = call-by-ref "?"(reference=w579, error in=w580, "Mode"=T51."Get Channel Names") -> (reference out=w581:refnum<vi>)  [unwired: 5 in, 1 out]
            n237 = Close Reference(reference=w581) -> ()  [unwired: 1 in, 1 out]
            n238 = event-data() -> ()  [unwired: 1 in, 5 out]
          }
          event "Plot Meas Chs": Mouse Down {
            n239 = event-data() -> ()  [unwired: 9 out]
            n240 = global read "Constants_global.vi" "EnFlo SW Folder"() -> (w593:path)
            n241 = Build Path(base path=w593, name or relative path=path "Anemometry/Utilities/Plot Meas channels.vi") -> (appended path=w584:path)
            n242 = Open VI Reference(vi path=w584) -> (vi reference=w587:refnum<vi>, error out=w585:errorcluster)  [unwired: 1 in, 4 out]
            n243 = property class="VI"(reference=w587, error in=w585, "Front Panel Window:Open"=TRUE) -> (reference out=w588:refnum<vi>, error out=w589:errorcluster)
            n244 = invoke class="VI" method="Run VI"(reference=w588, error in=w589, "Wait until done"=FALSE, "Auto Dispose Ref"=TRUE) -> (reference out=w590:refnum<vi>)  [unwired: 1 in, 4 out]
            n245 = Close Reference(reference=w590) -> ()  [unwired: 1 in, 1 out]
          }
          event "EnFlo Tun Display": Mouse Down? {
            n246 = event-data() -> ()  [unwired: 9 out]
            n247 = global read "Constants_global.vi" "EnFlo SW Folder"() -> (w605:path)
            n248 = Build Path(base path=w605, name or relative path=path "Anemometry/Utilities/EnFlo_Tunnel_Display.vi") -> (appended path=w601:path)
            n249 = Open VI Reference(vi path=w601) -> (vi reference=w600:refnum<vi>, error out=w599:errorcluster)  [unwired: 5 in]
            n250 = invoke class="VI" method="FP.Open"(reference=w600, error in=w599, "Activate"=TRUE ("Activate?"), "State"=T52."Standard") -> (reference out=w598:refnum<vi>, error out=w597:errorcluster)  [unwired: 1 in, 3 out]
            n251 = invoke class="VI" method="Run VI"(reference=w598, error in=w597, "Wait until done"=FALSE ("Wait Until Done"), "Auto Dispose Ref"=FALSE ("Wait until done")) -> (reference out=w602:refnum<vi>)  [unwired: 1 in, 4 out]
            n252 = Close Reference(reference=w602) -> ()  [unwired: 1 in, 1 out]
            n253 = event-data() -> ()  [unwired: 5 in, 1 out]
          }
          event Mouse Down? {
            n254 = event-data() -> ()  [unwired: 5 out]
            n255 = global read "Constants_global.vi" "EnFlo SW Folder"() -> (w607:path)
            n256 = Build Path(base path=w607, name or relative path=path "ADAM Client/ADAM client VIs/Set_Tunnel_Speed.vi") -> (appended path=w610:path)
            n257 = call "Open_Close_Front_Panel.ph.vi"("openWindow (T)"=TRUE ("Front Panel Window:Open"), "VI path"=w610) -> ()  [unwired: 1 in, 1 out]
            n258 = event-data() -> ()  [unwired: 1 in, 5 out]
          }
          event Mouse Down? {
            n259 = event-data() -> ()  [unwired: 5 out]
            n260 = global read "Constants_global.vi" "EnFlo SW Folder"() -> (w611:path)
            n261 = Build Path(base path=w611, name or relative path=path "ADAM Client/ADAM client VIs/Plot_Server_Data.vi") -> (appended path=w614:path)
            n262 = Open VI Reference(vi path=w614) -> (vi reference=w616:refnum<vi>, error out=w613:errorcluster)  [unwired: 1 in, 4 out]
            n263 = property class="VI"(reference=w616, error in=w613, "Front Panel Window:Open"=TRUE) -> (reference out=w617:refnum<vi>, error out=w618:errorcluster)
            n264 = invoke class="VI" method="Run VI"(reference=w617, error in=w618, "Wait until done"=FALSE, "Auto Dispose Ref"=TRUE) -> (reference out=w619:refnum<vi>)  [unwired: 1 in, 4 out]
            n265 = Close Reference(reference=w619) -> ()  [unwired: 1 in, 1 out]
            n266 = event-data() -> ()  [unwired: 1 in, 5 out]
          }
          event Mouse Down? {
            n267 = event-data() -> ()  [unwired: 5 out]
            n268 = global read "Constants_global.vi" "EnFlo SW Folder"() -> (w628:path)
            n269 = Build Path(base path=w628, name or relative path=path "ADAM Server/ADAM_scan_table.vi") -> (appended path=w626:path)
            n270 = Open VI Reference(vi path=w626) -> (vi reference=w629:refnum<vi>, error out=w630:errorcluster)  [unwired: 1 in, 4 out]
            n271 = property class="VI"(reference=w629, error in=w630) -> (reference out=w624:refnum<vi>, error out=w623:errorcluster, "Execution:State"=w631:T50)
            n272 = Equal?(x=w631, y=T50."Run top level" ("Execution:State")) -> (x = y?=w625:bool)
            n273 = case shown="False" w625 {
              tunnel: w624 -> [w636 w653]
              tunnel: w623 -> [w635 w652]
              tunnel: [w634 w653] -> w622
              tunnel: [w633 w652] -> _
              frame False {
                n274 = Two Button Dialog(message="Are you sure that you want to Run the ADAM Scan table on this machine?", 1:"Run" ("F button name (\"Cancel\")"), 2:"Cancel" ("T button name (\"OK\")")) -> (T button?=w637:bool)
                n275 = case shown="False" w637 {
                  tunnel: w636 -> [w644 w651]
                  tunnel: w635 -> [w643 w650]
                  tunnel: [w642 w651] -> w634
                  tunnel: [w641 w650] -> w633
                  frame False {
                    n276 = property class="VI"(reference=w644, error in=w643, "Front Panel Window:Open"=TRUE) -> (reference out=w648:refnum<vi>, error out=w647:errorcluster)
                    n277 = invoke class="VI" method="Run VI"(reference=w648, error in=w647, "Wait until done"=FALSE, "Auto Dispose Ref"=TRUE) -> (reference out=w642:refnum<vi>, error out=w641:errorcluster)  [unwired: 1 in, 3 out]
                  }
                  frame True {
                  }
                }
              }
              frame True {
              }
            }
            n278 = event-data() -> ()  [unwired: 1 in, 2 out]
            n279 = Close Reference(reference=w622) -> ()  [unwired: 1 in, 1 out]
          }
          event Mouse Down? {
            n280 = event-data() -> ()  [unwired: 5 out]
            n281 = global read "Constants_global.vi" "EnFlo SW Folder"() -> (w656:path)
            n282 = Build Path(base path=w656, name or relative path=path "ADAM Serial/Instrument drivers/Traverses/~subVIs/Read_Write_Trav_Config.vi") -> (appended path=w657:path)
            n283 = Build Path(base path=w656, name or relative path=path "ADAM Serial/Instrument drivers/Traverses/~subVIs/DriveConfigGlobal.vi") -> (appended path=w658:path)
            n284 = flat-sequence {
              tunnel: w658 -> [w659]
              tunnel: w657 -> [w661]
              frame #0 {
                n285 = call "Open_Close_Front_Panel.ph.vi"("openWindow (T)"=TRUE ("Front Panel Window:Open"), "VI path"=w659) -> ()  [unwired: 1 in, 1 out]
              }
              frame #1 {
                n286 = call "Open_Close_Front_Panel.ph.vi"("openWindow (T)"=TRUE ("Front Panel Window:Open"), "VI path"=w661) -> ()  [unwired: 1 in, 1 out]
              }
            }
            n287 = event-data() -> ()  [unwired: 1 in, 5 out]
          }
          event Mouse Down? {
            n288 = event-data() -> ()  [unwired: 5 out]
            n289 = global read "Constants_global.vi" "EnFlo SW Folder"() -> (w663:path)
            n290 = Build Path(base path=w663, name or relative path=path "Anemometry/Utilities/Hot_wire_Calculator.vi") -> (appended path=w666:path)
            n291 = call "Open_Close_Front_Panel.ph.vi"("openWindow (T)"=TRUE ("Front Panel Window:Open"), "VI path"=w666) -> ()  [unwired: 1 in, 1 out]
            n292 = event-data() -> ()  [unwired: 1 in, 5 out]
          }
          event "Show Manual Sync": Mouse Down {
            n293 = event-data() -> ()  [unwired: 9 out]
            n294 = global read "Constants_global.vi" "EnFlo SW Folder"() -> (w667:path)
            n295 = Build Path(base path=w667, name or relative path=path "Anemometry/Utilities/EnFlo_Data_Sync_Manual.vi") -> (appended path=w670:path)
            n296 = call "Open_Close_Front_Panel.ph.vi"("openWindow (T)"=TRUE ("Front Panel Window:Open"), "VI path"=w670) -> ()  [unwired: 1 in, 1 out]
          }
          event "Plot_FFID_Calibs.vi": Mouse Down {
            n297 = event-data() -> ()  [unwired: 9 out]
            n298 = global read "Constants_global.vi" "EnFlo SW Folder"() -> (w680:path)
            n299 = Build Path(base path=w680, name or relative path=path "ADAM Client/ADAM client VIs/Plot_FFID_Calibs.vi") -> (appended path=w671:path)
            n300 = Open VI Reference(vi path=w671) -> (vi reference=w674:refnum<vi>, error out=w672:errorcluster)  [unwired: 1 in, 4 out]
            n301 = property class="VI"(reference=w674, error in=w672, "Front Panel Window:Open"=TRUE) -> (reference out=w675:refnum<vi>, error out=w676:errorcluster)
            n302 = invoke class="VI" method="Run VI"(reference=w675, error in=w676, "Wait until done"=FALSE, "Auto Dispose Ref"=TRUE) -> (reference out=w677:refnum<vi>)  [unwired: 1 in, 4 out]
            n303 = Close Reference(reference=w677) -> ()  [unwired: 1 in, 1 out]
          }
          event "Display Bad Trav Points": Mouse Down? {
            n304 = event-data() -> ()  [unwired: 9 out]
            n305 = global read "Constants_global.vi" "EnFlo SW Folder"() -> (w691:path)
            n306 = Build Path(base path=w691, name or relative path=path "Anemometry/Anemometry Sub Vis/Gen Trav/Display_Bad_Positions.vi") -> (appended path=w682:path)
            n307 = Open VI Reference(vi path=w682) -> (vi reference=w685:refnum<vi>, error out=w683:errorcluster)  [unwired: 1 in, 4 out]
            n308 = property class="VI"(reference=w685, error in=w683, "Front Panel Window:Open"=TRUE) -> (reference out=w686:refnum<vi>, error out=w687:errorcluster)
            n309 = invoke class="VI" method="Run VI"(reference=w686, error in=w687, "Wait until done"=FALSE, "Auto Dispose Ref"=TRUE) -> (reference out=w688:refnum<vi>)  [unwired: 1 in, 4 out]
            n310 = Close Reference(reference=w688) -> ()  [unwired: 1 in, 1 out]
            n311 = event-data() -> ()  [unwired: 2 in, 1 out]
          }
          event "Move Mirror": Mouse Down? {
            n312 = event-data() -> ()  [unwired: 9 out]
            n313 = global read "Constants_global.vi" "EnFlo SW Folder"() -> (w699:path)
            n314 = Build Path(base path=w699, name or relative path=path "Anemometry/Anemometry Sub Vis/Gen Trav/Move_LDA_Mirror.vi") -> (appended path=w695:path)
            n315 = Open VI Reference(vi path=w695) -> (vi reference=w698:refnum<vi>, error out=w696:errorcluster)  [unwired: 1 in, 4 out]
            n316 = property class="VI"(reference=w698, error in=w696, "Front Panel Window:Open"=TRUE) -> (reference out=w694:refnum<vi>, error out=w693:errorcluster)
            n317 = Close Reference(reference=w694, error in (no error)=w693) -> ()  [unwired: 1 out]
            n318 = event-data() -> ()  [unwired: 2 in, 1 out]
          }
          event "SaveFPs": Mouse Up {
            n319 = event-data() -> ()  [unwired: 9 out]
            n320 = call "GetLocnsAndSave.vi"() -> ()  [unwired: 12 in]
          }
          event "HierarchyHealthcheck": Mouse Up {
            n321 = event-data() -> ()  [unwired: 9 out]
            n322 = call "CheckHierarchyStatus.vi"() -> ()  [unwired: 12 in]
          }
          event "ResetFPs": Mouse Up {
            n323 = event-data() -> ()  [unwired: 9 out]
            n324 = call "ResetFPlocns.vi"() -> ()  [unwired: 12 in]
          }
          event "Beam Check Positions": Mouse Down {
            n325 = event-data() -> ()  [unwired: 9 out]
            n326 = global read "Constants_global.vi" "EnFlo SW Folder"() -> (w703:path)
            n327 = Build Path(base path=w703, name or relative path=path "Anemometry/Anemometry Sub Vis/LDA/Input_Beam_Check_Locations.vi") -> (appended path=w701:path)
            n328 = call "Open_Close_Front_Panel.ph.vi"("openWindow (T)"=TRUE ("Front Panel Window:Open"), "VI path"=w701) -> ()  [unwired: 1 in, 1 out]
          }
          event "Beam Power Meter": Mouse Down {
            n329 = event-data() -> ()  [unwired: 9 out]
            n330 = global read "Constants_global.vi" "EnFlo SW Folder"() -> (w707:path)
            n331 = Build Path(base path=w707, name or relative path=path "ADAM Serial/Instrument drivers/PM100D/PM100D_Read_ph.vi") -> (appended path=w705:path)
            n332 = call "Open_Close_Front_Panel.ph.vi"("openWindow (T)"=TRUE ("Front Panel Window:Open"), "VI path"=w705) -> ()  [unwired: 1 in, 1 out]
          }
          event Mouse Down? {
            n333 = event-data() -> ()  [unwired: 5 out]
            n334 = global read "Constants_global.vi" "EnFlo SW Folder"() -> (w709:path)
            n335 = Build Path(base path=w709, name or relative path=path "Anemometry/Utilities/Hydrosonic_Manual.vi") -> (appended path=w712:path)
            n336 = call "Open_Close_Front_Panel.ph.vi"("openWindow (T)"=TRUE ("Front Panel Window:Open"), "VI path"=w712) -> ()  [unwired: 1 in, 1 out]
            n337 = event-data() -> ()  [unwired: 1 in, 5 out]
          }
          event "Mult Trav Move": Value Change {
            n338 = event-data() -> ()  [unwired: 7 out]
            n339 = global read "Constants_global.vi" "EnFlo SW Folder"() -> (w713:path)
            n340 = Build Path(base path=w713, name or relative path=path "Anemometry/Multi_Trav_Move.vi") -> (appended path=w716:path)
            n341 = call "Open_Close_Front_Panel.ph.vi"("openWindow (T)"=TRUE ("Front Panel Window:Open"), "VI path"=w716) -> ()  [unwired: 1 in, 1 out]
          }
          event "Top Level Traverse": Mouse Down {
            n342 = event-data() -> ()  [unwired: 9 out]
            n343 = global read "Constants_global.vi" "EnFlo SW Folder"() -> (w717:path)
            n344 = Build Path(base path=w717, name or relative path=path "Anemometry/Utilities/Top_Level_Move_Traverse.vi") -> (appended path=w720:path)
            n345 = call "Open_Close_Front_Panel.ph.vi"("openWindow (T)"=TRUE ("Front Panel Window:Open"), "VI path"=w720) -> ()  [unwired: 1 in, 1 out]
          }
          event "Post_Pro_Results_Hierarchy": Mouse Down {
            n346 = event-data() -> ()  [unwired: 9 out]
            n347 = global read "Constants_global.vi" "EnFlo SW Folder"() -> (w721:path)
            n348 = Build Path(base path=w721, name or relative path=path "Anemometry/Utilities/Post_Pro_Results_Hierarchy.vi") -> (appended path=w724:path)
            n349 = call "Open_Close_Front_Panel.ph.vi"("openWindow (T)"=TRUE ("Front Panel Window:Open"), "VI path"=w724) -> ()  [unwired: 1 in, 1 out]
          }
          event Mouse Down? {
            n350 = event-data() -> ()  [unwired: 5 out]
            n351 = global read "Constants_global.vi" "EnFlo SW Folder"() -> (w725:path)
            n352 = Build Path(base path=w725, name or relative path=path "Anemometry/Utilities/Preference_Panel.vi") -> (appended path=w733:path)
            n353 = Open VI Reference(type specifier VI Refnum (for type only)=refnum<vi> refnum, vi path=w733) -> (vi reference=w727:refnum<vi>, error out=w728:errorcluster)  [unwired: 1 in, 3 out]
            n354 = property class="VI Interface Type 6"(reference=w727, error in=w728, "Front Panel Window:Open"=TRUE) -> (reference out=w730:refnum<vi>, error out=w731:errorcluster)
            n355 = call-by-ref "?"(reference=w730, error in=w731, "Mode"=Preference_Mode."Load, Edit then Save") -> (reference out=w732:refnum<vi>)  [unwired: 1 out]
            n356 = Close Reference(reference=w732) -> ()  [unwired: 1 in, 1 out]
            n357 = event-data("Discard?"=TRUE) -> ()  [unwired: 1 in, 4 out]
          }
          event Mouse Down? {
            n358 = event-data() -> ()  [unwired: 5 out]
            n359 = global read "Constants_global.vi" "EnFlo SW Folder"() -> (w739:path)
            n360 = Build Path(base path=w739, name or relative path=path "ADAM Client/Sub VIs/Gas_Setup.vi") -> (appended path=w746:path)
            n361 = Open VI Reference(type specifier VI Refnum (for type only)=refnum<vi> refnum, vi path=w746) -> (vi reference=w742:refnum<vi>, error out=w743:errorcluster)  [unwired: 1 in, 3 out]
            n362 = property class="VI Interface Type 7"(reference=w742, error in=w743, "Front Panel Window:Open"=TRUE) -> (reference out=w747:refnum<vi>, error out=w745:errorcluster)
            n363 = call-by-ref "?"(reference=w747, error in=w745) -> (reference out=w737:refnum<vi>)  [unwired: 9 in, 1 out]
            n364 = Close Reference(reference=w737) -> ()  [unwired: 1 in, 1 out]
            n365 = event-data("Discard?"=TRUE) -> ()  [unwired: 1 in, 4 out]
          }
          event Mouse Down? {
            n366 = event-data() -> ()  [unwired: 5 out]
            n367 = global read "Constants_global.vi" "EnFlo SW Folder"() -> (w750:path)
            n368 = Build Path(base path=w750, name or relative path=path "ADAM Client/Sub VIs/User_Metadata.vi") -> (appended path=w757:path)
            n369 = Open VI Reference(type specifier VI Refnum (for type only)=refnum<vi> refnum, vi path=w757) -> (vi reference=w753:refnum<vi>, error out=w754:errorcluster)  [unwired: 1 in, 3 out]
            n370 = property class="VI Interface Type 7"(reference=w753, error in=w754, "Front Panel Window:Open"=TRUE) -> (reference out=w758:refnum<vi>, error out=w756:errorcluster)
            n371 = call-by-ref "?"(reference=w758, error in=w756) -> (reference out=w748:refnum<vi>)  [unwired: 9 in, 1 out]
            n372 = Close Reference(reference=w748) -> ()  [unwired: 1 in, 1 out]
            n373 = event-data("Discard?"=TRUE) -> ()  [unwired: 1 in, 4 out]
          }
          event Mouse Down? {
            n374 = event-data() -> ()  [unwired: 5 out]
            n375 = global read "Constants_global.vi" "EnFlo SW Folder"() -> (w763:path)
            n376 = Build Path(base path=w763, name or relative path=path "ADAM Client/Sub VIs/EnFlo_Tunnel_Setup.vi") -> (appended path=w766:path)
            n377 = Open VI Reference(type specifier VI Refnum (for type only)=refnum<vi> refnum, vi path=w766) -> (vi reference=w761:refnum<vi>, error out=w760:errorcluster)  [unwired: 1 in, 3 out]
            n378 = call-by-ref "?"(reference=w761, error in=w760) -> (reference out=w762:refnum<vi>)  [unwired: 9 in, 1 out]
            n379 = Close Reference(reference=w762) -> ()  [unwired: 1 in, 1 out]
            n380 = event-data("Discard?"=TRUE) -> ()  [unwired: 1 in, 4 out]
          }
          event Mouse Down? {
            w780 = TRUE  # Show Panel?
            n381 = event-data() -> ()  [unwired: 5 out]
            n382 = global read "Preference_global.vi" "Use New Collision Code"() -> (w771:bool)
            n383 = global read "Constants_global.vi" "EnFlo SW Folder"() -> (w776:path)
            n384 = Select(t=path "Anemometry/Anemometry Sub Vis/Gen Trav/Traverse_Space_for new collision code.vi", s=w771, f=path "Anemometry/Anemometry Sub Vis/Gen Trav/Traverse_Space.vi") -> (s? t:f=w768:path)
            n385 = Build Path(base path=w776, name or relative path=w768) -> (appended path=w778:path)
            n386 = global read "Trav_pos_global.vi" "Default Traverse Setup"() -> (w772:string)
            n387 = Open VI Reference(type specifier VI Refnum (for type only)=refnum<vi> refnum, vi path=w778) -> (vi reference=w779:refnum<vi>, error out=w773:errorcluster)  [unwired: 1 in, 3 out]
            n388 = call-by-ref "?"(reference=w779, error in=w773, "Simulate/Run"=User_Specific_mode."Check VI only", "Show Panel?"=w780, "Traverse Setup"=w772) -> (reference out=w774:refnum<vi>)  [unwired: 7 in, 2 out]
            n389 = Close Reference(reference=w774) -> ()  [unwired: 1 in, 1 out]
            n390 = event-data("Discard?"=TRUE) -> ()  [unwired: 1 in, 4 out]
          }
          event Mouse Down? {
            n391 = event-data() -> ()  [unwired: 5 out]
            n392 = global read "Constants_global.vi" "EnFlo SW Folder"() -> (w782:path)
            n393 = Build Path(base path=w782, name or relative path=path "Anemometry/Anemometry Sub Vis/Traverse vi's/EnFlo Tunnel specific/Check_EnFlo_Arm.vi") -> (appended path=w784:path)
            n394 = call "Open_Close_Front_Panel.ph.vi"("openWindow (T)"=TRUE ("Front Panel Window:Open"), "VI path"=w784) -> ()  [unwired: 1 in, 1 out]
            n395 = event-data() -> ()  [unwired: 1 in, 2 out]
          }
          event Mouse Down? {
            n396 = event-data() -> ()  [unwired: 5 out]
            n397 = global read "Constants_global.vi" "EnFlo SW Folder"() -> (w792:path)
            n398 = Build Path(base path=w792, name or relative path=path "Anemometry/Anemometry Sub Vis/Gen Trav/3D_Traverse_move.vi") -> (appended path=w789:path)
            n399 = Strip Path(path=w789) -> (name=w788:string)  [unwired: 1 out]
            n400 = Open VI Reference(vi path=w788) -> (vi reference=w790:refnum<vi>, error out=w791:errorcluster)  [unwired: 1 in, 4 out]
            n401 = property class="VI"(reference=w790, error in=w791) -> (reference out=w786:refnum<vi>, error out=w785:errorcluster, "Front Panel Window:Open"=w787:bool)
            n402 = case shown="False" w787 {
              tunnel: w789 -> [w797 _]
              tunnel: w786 -> [_ w812]
              tunnel: w785 -> [_ w811]
              frame False {
                w794 = TRUE  # Route Checking?
                w796 = TRUE  # Last Part of Move?
                n403 = global read "Trav_pos_global.vi" "Work in Tunnel Coordinates?"() -> (w806:T59)
                n404 = global read "Trav_pos_global.vi" "Default Traverse Setup"() -> (w804:string)
                n405 = Open VI Reference(type specifier VI Refnum (for type only)=refnum<vi> refnum, vi path=w797) -> (vi reference=w801:refnum<vi>, error out=w802:errorcluster)  [unwired: 1 in, 3 out]
                n406 = property class="VI Interface Type 8"(reference=w801, error in=w802, "Front Panel Window:Open"=TRUE) -> (reference out=w798:refnum<vi>, error out=w799:errorcluster)
                n407 = call-by-ref "?"(reference=w798, error in=w799, "Mode"=Trav_mode."Read traverse position", "Extra command String"="", "Work in Tunnel Coordinates"=w806, "Simulate/Run"=User_Specific_mode."Run VI", "Route Checking?"=w794, "Traverse name"=w804, "Last Part of Move?"=w796) -> (reference out=w803:refnum<vi>)  [unwired: 9 in, 5 out]
                n408 = Close Reference(reference=w803) -> ()  [unwired: 1 in, 1 out]
              }
              frame True {
                n409 = property class="VI"(reference=w812, error in=w811, "Front Panel Window:Open"=TRUE) -> (reference out=w810:refnum<vi>)  [unwired: 1 out]
                n410 = Close Reference(reference=w810) -> ()  [unwired: 1 in, 1 out]
              }
            }
            n411 = event-data() -> ()  [unwired: 1 in, 5 out]
          }
          event Mouse Down? {
            n412 = event-data() -> ()  [unwired: 5 out]
            n413 = Open VI Reference(vi path="Multi_Run_Prog.vi") -> (vi reference=w818:refnum<vi>, error out=w817:errorcluster)  [unwired: 1 in, 4 out]
            n414 = property class="VI"(reference=w818, error in=w817, "Front Panel Window:Open"=TRUE) -> (reference out=w816:refnum<vi>, error out=w813:errorcluster)
            n415 = Close Reference(reference=w816, error in (no error)=w813) -> (error out=w814:errorcluster)
            n416 = Unbundle By Name(w814) -> ("status"=w820:bool)
            n417 = case shown="True" w820 {
              frame False {
              }
              frame True {
                n418 = global read "Constants_global.vi" "EnFlo SW Folder"() -> (w828:path)
                n419 = call "Setup_Filepath.vi"("Setup File Type"=Setup_Filetype."General", "Filename in"="Multi_Run_Filename.txt" ("name or relative path")) -> ("Filename Out"=w822:path)  [unwired: 1 out]
                n420 = Build Path(base path=w828, name or relative path=path "Anemometry/Multi_Run_Prog.vi") -> (appended path=w827:path)
                n421 = call "Read Characters with check.vi"("file (use dialog)"=w822) -> ("Read String"=w821:string)  [unwired: 1 in, 1 out]
                n422 = String To Path(string=w821) -> (path=w825:path)
                n423 = call "Does_file_exist_(simple).vi"("Pathname"=w825) -> ("exists?"=w826:bool)
                n424 = case shown="True" w826 {
                  tunnel: w827 -> [w830 w841]
                  tunnel: w825 -> [_ w839]
                  frame False {
                    n425 = call "Open_Close_Front_Panel.ph.vi"("openWindow (T)"=TRUE ("Front Panel Window:Open"), "VI path"=w830) -> ()  [unwired: 1 in, 1 out]
                  }
                  frame True {
                    n426 = Open VI Reference(type specifier VI Refnum (for type only)=refnum<vi> refnum, vi path=w841) -> (vi reference=w838:refnum<vi>, error out=w837:errorcluster)  [unwired: 1 in, 3 out]
                    n427 = property class="VI Interface Type 9"(reference=w838, error in=w837, "Front Panel Window:Open"=TRUE) -> (reference out=w835:refnum<vi>, error out=w836:errorcluster)
                    n428 = call-by-ref "?"(reference=w835, error in=w836, "Command filename"=w839, "Mode"=T55."Load Command File" ("Setup mode")) -> (reference out=w834:refnum<vi>)  [unwired: 17 in, 2 out]
                    n429 = Close Reference(reference=w834) -> ()  [unwired: 1 in, 1 out]
                  }
                }
              }
            }
            n430 = event-data() -> ()  [unwired: 1 in, 5 out]
          }
          event Mouse Down? {
            w843 = "Calibration.vi" ("name or relative path")
            n431 = event-data() -> ()  [unwired: 5 out]
            n432 = global read "Constants_global.vi" "EnFlo SW Folder"() -> (w849:path)
            n433 = Open VI Reference(vi path=w843) -> (vi reference=w847:refnum<vi>, error out=w846:errorcluster)  [unwired: 1 in, 4 out]
            n434 = Build Path(base path=w849, name or relative path="Anemometry") -> (appended path=w852:path)
            n435 = property class="VI"(reference=w847, error in=w846, "Front Panel Window:Open"=TRUE) -> (reference out=w844:refnum<vi>, error out=w845:errorcluster)
            n436 = Build Path(base path=w852, name or relative path=w843) -> (appended path=w850:path)
            n437 = Close Reference(reference=w844, error in (no error)=w845) -> (error out=w842:errorcluster)
            n438 = Unbundle By Name(w842) -> ("status"=w851:bool)
            n439 = case shown="True" w851 {
              tunnel: w850 -> [_ w854]
              tunnel: w842 -> [_ _]
              frame False {
              }
              frame True {
                n440 = stacked-sequence {
                  seq-local: [w861 _] -> [_ w867]
                  tunnel: w854 -> [_ w868]
                  frame #0 {
                    n441 = call "Setup_Filepath.vi"("Setup File Type"=Setup_Filetype."Calibration Setups", "Filename in"="Current_Setup.xls") -> ("Filename Out"=w856:path)  [unwired: 1 out]
                    n442 = call "Read Characters with check.vi"("file (use dialog)"=w856) -> ("Read String"=w855:string)  [unwired: 1 in, 1 out]
                    n443 = Format Into String(format string="Calibration Setup File   %s", w856) -> (resulting string=w859:string)  [unwired: 2 in, 1 out]
                    n444 = call "Get_string_subset.vi"("String Name"=w859, "String to split"=w855, "File Label"="Raw data header") -> ("Output string"=w863:string)  [unwired: 1 in, 1 out]
                    n445 = call "Get_Characters_from_string.vi"("Input string"=w863, "Variable name"="Calib filename") -> ("Value"=w862:string)  [unwired: 1 in, 1 out]
                    n446 = call "String_to_Pathname.vi"("Input String"=w862) -> ("path"=w861:path)
                  }
                  frame #1 {
                    n447 = call "Does_file_exist_(simple).vi"("Pathname"=w867) -> ("exists?"=w866:bool)
                    n448 = case shown="True" w866 {
                      tunnel: w868 -> [w869 w883]
                      tunnel: w867 -> [_ w877]
                      frame False {
                        n449 = call "Open_Close_Front_Panel.ph.vi"("openWindow (T)"=TRUE ("Front Panel Window:Open"), "VI path"=w869) -> ()  [unwired: 1 in, 1 out]
                      }
                      frame True {
                        w875 = TRUE ("Front Panel Window:Open")
                        n450 = Open VI Reference(type specifier VI Refnum (for type only)=refnum<vi> refnum, vi path=w883) -> (vi reference=w881:refnum<vi>, error out=w876:errorcluster)  [unwired: 1 in, 3 out]
                        n451 = property class="VI Interface Type 10"(reference=w881, error in=w876, "Front Panel Window:Open"=w875, "Front Panel Window:Auto Center (Deprecated)"=w875) -> (reference out=w880:refnum<vi>, error out=w879:errorcluster)
                        n452 = call-by-ref "?"(reference=w880, error in=w879, "Mode"=Calib_mode."Setup Front Panel", "Calib file"=w877) -> (reference out=w873:refnum<vi>, error out=w872:errorcluster)  [unwired: 15 in, 3 out]
                        n453 = property class="VI Interface Type 10"(reference=w873, error in=w872, "Front Panel Window:Auto Center (Deprecated)"=FALSE ("Front Panel Window:Auto Center")) -> (reference out=w871:refnum<vi>)  [unwired: 1 out]
                        n454 = Close Reference(reference=w871) -> ()  [unwired: 1 in, 1 out]
                      }
                    }
                  }
                }
              }
            }
            n455 = event-data() -> ()  [unwired: 1 in, 5 out]
          }
          event "stop": Mouse Up {
            n456 = event-data() -> ()  [unwired: 9 out]
            n457 = Open VI Reference(vi path="CPP_Launcher.vi") -> (vi reference=w887:refnum<vi>, error out=w890:errorcluster)  [unwired: 5 in]
            n458 = invoke class="VI" method="Abort VI"(reference=w887, error in=w890) -> (reference out=w889:refnum<vi>, error out=w888:errorcluster)  [unwired: 1 in, 1 out]
            n459 = Close Reference(reference=w889, error in (no error)=w888) -> (error out=w886:errorcluster)
            n460 = call "Synchronize Data Flow.vim"("input 4"=w886, "input 1"=TRUE ("stop? (T)")) -> ("output 1"=w884:bool)  [unwired: 2 in, 3 out]
            n461 = Stop(stop? (T)=w884) -> ()
          }
          event Panel Close? {
            n462 = event-data() -> ("VIRef"=w893:refnum<vi>)  [unwired: 4 out]
            n463 = Open VI Reference(vi path="CPP_Launcher.vi") -> (vi reference=w895:refnum<vi>, error out=w898:errorcluster)  [unwired: 5 in]
            n464 = invoke class="VI" method="Abort VI"(reference=w895, error in=w898) -> (reference out=w897:refnum<vi>, error out=w896:errorcluster)  [unwired: 1 in, 1 out]
            n465 = Close Reference(reference=w897, error in (no error)=w896) -> (error out=w894:errorcluster)
            n466 = call "Synchronize Data Flow.vim"("input 4"=w894, "input 1"=w893) -> ("output 1"=w892:refnum<vi>)  [unwired: 2 in, 3 out]
            n467 = invoke class="VI" method="FP.Close"(reference=w892) -> ()  [unwired: 2 in, 3 out]
            n468 = event-data() -> ()  [unwired: 2 in, 1 out]
          }
          event "Rig_Control": Value Change {
            n469 = event-data() -> ("OldVal"=w901:cluster{"Ch Name":string, "Boolean":bool}[], "NewVal"=w900:cluster{"Ch Name":string, "Boolean":bool}[])  [unwired: 5 out]
            n470 = for {
              tunnel: w901 -> [w907] mode=indexing
              tunnel: w900 -> [w906] mode=indexing
              n471 = Unbundle By Name(w907) -> ("Ch Name"=w904:string, "Boolean"=w905:bool)
              n472 = Unbundle By Name(w906) -> ("Boolean"=w903:bool)  [unwired: 1 out]
              n473 = Not Equal?(x=w905, y=w903) -> (x != y?=w902:bool)
              n474 = case shown="True" w902 {
                tunnel: w904 -> [_ w908]
                tunnel: w903 -> [_ w914]
                frame False {
                }
                frame True {
                  n475 = call "Get_Current_Scan_client.vi"("singleChannel"=w908) -> ("Ch Description Array"=w913:T42[])  [unwired: 1 in, 3 out]
                  n476 = Index Array(array=w913) -> (element=w909:T42)  [unwired: 1 in]
                  n477 = Unbundle By Name(w909) -> ("Type"=w912:T43)
                  n478 = Equal?(x=T43 "Count Down Timer" ("Type"), y=w912) -> (x = y?=w910:bool)
                  n479 = case shown="True" w914 {
                    tunnel: ["On" "Off"] -> w916
                    tunnel: [w926 w934] -> w915
                    tunnel: w910 -> [w927 w935]
                    tunnel: w909 -> [w925 w933]
                    frame True {
                      n480 = Unbundle By Name(w925) -> ("A"=w924:dbl)
                      n481 = Absolute Value(x=w924) -> (abs(x)=w923:dbl)
                      n482 = Select(t=w923, s=w927, f=1.0) -> (s? t:f=w926:dbl)
                    }
                    frame False {
                      n483 = Unbundle By Name(w933) -> ("B"=w932:dbl)
                      n484 = Absolute Value(x=w932) -> (abs(x)=w931:dbl)
                      n485 = Negate(x=w931) -> (-x=w930:dbl)
                      n486 = Select(t=w930, s=w935, f=0.0) -> (s? t:f=w934:dbl)
                    }
                  }
                  n487 = Format Into String(format string="Are you sure you want to turn %s %s?", w908, w916) -> (resulting string=w921:string)  [unwired: 2 in, 1 out]
                  n488 = Format Into String(format string="Make  %s  %s", w908, w916) -> (resulting string=w917:string)  [unwired: 2 in, 1 out]
                  n489 = Two Button Dialog(message=w921, 1:w917, 2:"Cancel" ("T button name (\"OK\")")) -> (T button?=w919:bool)
                  n490 = case shown="False" w919 {
                    tunnel: w908 -> [w939 _]
                    tunnel: w915 -> [w938 _]
                    frame False {
                      n491 = Build Array(w939) -> (w940:string[])
                      n492 = Build Array(w938) -> (w941:dbl[])
                      n493 = call "ASYNC_Adam_client.vi"("Values"=w941, "Channel Names"=w940) -> ()  [unwired: 1 in, 2 out]
                    }
                    frame True {
                    }
                  }
                }
              }
            }
          }
          event "Edit Channel Interactive": Mouse Up {
            w942 = TRUE ("runVI (F)")
            n494 = event-data() -> ()  [unwired: 2 out]
            n495 = global read "Constants_global.vi" "EnFlo SW Folder"() -> (w943:path)
            n496 = Build Path(base path=w943, name or relative path=path "ADAM Client/ADAM client VIs/EditServerChannelInteractive.vi") -> (appended path=w945:path)
            n497 = call "Open_Close_Front_Panel.ph.vi"("runVI (F)"=w942, "openWindow (T)"=w942, "VI path"=w945) -> ()  [unwired: 1 out]
          }
          event "changelog": Mouse Up {
            n498 = event-data() -> ()  [unwired: 2 out]
            n499 = global read "Constants_global.vi" "EnFlo SW Folder"() -> (w946:path)
            n500 = Build Path(base path=w946, name or relative path=path "Anemometry/Utilities/SW_Update_Tool/makeChangelogSVN.vi") -> (appended path=w949:path)
            n501 = call "Open_Close_Front_Panel.ph.vi"("openWindow (T)"=TRUE ("Front Panel Window:Open"), "VI path"=w949) -> ()  [unwired: 1 in, 1 out]
          }
        }
        "Numeric" <- w386
      }
      n502 = while {
        shift-left: _ -> [w952]
        shift-right: [w953] -> _
        shift-left: "Initialise" -> [w951]
        shift-right: [w954] -> _
        i -> [w950]
        stop <- TRUE continue-if-true
        # "Remote call launcher and Global retainer"
        n503 = case shown="\"No match\", Default" w951 {
          selector: w951 -> [w956 _ _ _ _ _ _ _ _ _ _]
          tunnel: ["End" "Initialise" "Wait for call remote sub vi occurrence" "Check type of VI to launch" w978 "Wait until remote sub vi is opened" "Update opened vis array" "Update opened vis array" "Update opened vis array" "Wait until remote sub vi is opened" "Wait for call remote sub vi occurrence"] -> w954
          tunnel: [w957 w966 w969 errorcluster {"status"=FALSE, "code"=0, "source"=""} ("error out") w974 w991 w1023 w1040 w1055 w1095 w1115] -> w953
          tunnel: w952 -> [w957 w966 w969 _ w974 w991 _ _ _ w1095 w1115]
          tunnel: w950 -> [_ _ _ _ _ _ _ _ _ _ _]
          frame "No match", Default {
            n504 = call "Case not matched.vi"("Case Name not Matched"=w956) -> ()
          }
          frame "Never run" {
            # "This keeps the Coherent global and DLL reference alive even after all associated vi's are closed and the Hub is stopped (but not closed, that really is game over....)"
            # "These globals are here to make sure they stay in memory\nafter \"Preference Panel\" has finished running"
            n505 = call "Connect_to_BSA_F60.vi"("BSA IP Number"="", "Force Reconnect"=FALSE) -> ()  [unwired: 2 out]
            n506 = call "Email_With_Log.vi"() -> ()  [unwired: 4 in, 3 out]
            n507 = call "Overhead_Factor.vi"() -> ()  [unwired: 4 in, 1 out]
            n508 = call "Remember_value.vi"() -> ()  [unwired: 3 in, 1 out]
            n509 = call "Output_Trav_Pos.vi"() -> ()  [unwired: 5 in, 1 out]
            n510 = call "Read_Write_Local_table.vi"() -> ()  [unwired: 3 in, 3 out]
            n511 = global read "Trav_pos_global.vi" "Dummy Measurement?"() -> (→"Dummy Measurement":bool)
            n512 = global read "PWAtasksGLOBAL.vi" "PWA No. of Samples"() -> (→"PWA No. of Samples":i32)
            n513 = global read "Preference_global.vi" "Rig Setup"() -> (→"Rig Name":string)
            n514 = call "Get DLL version.vi"() -> ()  [unwired: 3 out]
            n515 = global read "Constants_global.vi" "All_Users"() -> (→"All Users":path)
          }
          frame "Initialise" {
            "Iterations" <- 0 ("Iterations")
          }
          frame "Wait for call remote sub vi occurrence" {
            n516 = global read "Dynamic_call_global.ph.vi" "Call Remote Subvi"() -> (w972:refnum<k4>)
            n517 = Wait on Occurrence(2:w972) -> ()  [unwired: 3 out]
          }
          frame "Check type of VI to launch" {
            n518 = global read "Dynamic_call_global.ph.vi" "VI name to launch"() -> (w976:string)
            n519 = Match Pattern(string=w976, regular expression=";") -> (before substring=w973:string, after substring=w975:string)  [unwired: 3 out]
            n520 = case shown="\"Open Analogue Input VI\"" w973 {
              selector: w973 -> [_ _ _ w986]
              tunnel: ["Open vi" "Open application reference" "Open Analogue input server" w986] -> w978
              tunnel: [w981 w983 w985 w987] -> w977
              tunnel: w976 -> [w981 _ _ _]
              tunnel: w975 -> [_ w983 w985 w987]
              frame "Other", Default {
              }
              frame "Open Application Reference" {
              }
              frame "Open Analogue Input VI" {
              }
              frame "Open LDA PWA & An" {
              }
            }
            "VI Name" <- w977
          }
          frame "Open application reference" {
            n521 = local read "VI Name"() -> (w992:string)
            n522 = call "App_Ref_Global.vi"("Mode"=App_Global."Read Global") -> ("Output Array"=w998:T60[])  [unwired: 1 in, 1 out]
            n523 = Match Pattern(string=w992, regular expression=";") -> (before substring=w1000:string, after substring=w1001:string)  [unwired: 3 out]
            n524 = Decimal String To Number(string=w1001) -> (number=w1002:i32)  [unwired: 3 out]
            n525 = To Unsigned Long Integer(number=w1002) -> (unsigned 32bit integer=w999:u32)
            n526 = Open Application Reference(10:w999, 11:w1000) -> (0:w993:errorcluster, 3:w997:refnum<vi>)  [unwired: 1 in, 1 out]
            n527 = global write "Dynamic_call_global.ph.vi" "Error Cluster"(w993) -> ()
            n528 = for {
              tunnel: w998 -> [w1006] mode=indexing
              tunnel: w992 -> [w1009]
              tunnel: w997 -> [w1008]
              tunnel: [w1010] -> w996 mode=indexing
              tunnel: [w1007] -> w988 mode=indexing if=w1005
              n529 = Unbundle By Name(w1006) -> ("Server IP & Port No"=w1011:string)
              n530 = Equal?(x=w1011, y=w1009) -> (x = y?=w1004:bool)
              n531 = case shown="False" w1004 {
                tunnel: w1008 -> [_ w1015]
                tunnel: [w1012 w1014] -> w1010
                tunnel: w1006 -> [w1012 w1013]
                frame False {
                }
                frame True {
                  n532 = Bundle By Name(cluster=w1013, "Application reference"=w1015) -> (w1014:T60)
                }
              }
              n533 = Bundle By Name(cluster=w1006, "Server IP & Port No"=w1009, "Application reference"=w1008) -> (w1007:T60)
              n534 = Not(x=w1004) -> (.not. x?=w1005:bool)
            }
            n535 = Build Array (concatenate)(w996, w988) -> (w989:T60[])
            n536 = call "App_Ref_Global.vi"("Input Array"=w989, "Mode"=App_Global."Write to Global") -> ()  [unwired: 2 out]
          }
          frame "Open Analogue input server" {
            n537 = local read "VI Name"() -> (w1020:string)
            n538 = call "Get_link_info.vi"("VI Name"=w1020) -> ("Application reference"=w1018:refnum<vi>, "Path name"=w1017:path, "Local Call?"=w1019:bool)  [unwired: 2 out]
            n539 = global read "Dynamic_call_global.ph.vi" "Analogue Input"() -> (w1022:refnum<vi>)
            n540 = case shown="False" w1019 {
              tunnel: w1022 -> [w1028 w1032]
              tunnel: [w1024 w1031] -> w1021
              tunnel: [w1027 w1030] -> w1023
              tunnel: w1020 -> [w1026 _]
              tunnel: w1018 -> [w1025 _]
              tunnel: w1017 -> [_ w1029]
              frame False {
                n541 = Open VI Reference(type specifier VI Refnum (for type only)=w1028, application reference (local)=w1025, vi path=w1026) -> (vi reference=w1024:refnum<vi>, error out=w1027:errorcluster)  [unwired: 1 in, 2 out]
              }
              frame True {
                n542 = Open VI Reference(type specifier VI Refnum (for type only)=w1032, vi path=w1029) -> (vi reference=w1031:refnum<vi>, error out=w1030:errorcluster)  [unwired: 1 in, 3 out]
              }
            }
            n543 = global write "Dynamic_call_global.ph.vi" "Analogue Input"(w1021) -> ()
          }
          frame "Open LDA PWA & An" {
            n544 = local read "VI Name"() -> (w1037:string)
            n545 = call "Get_link_info.vi"("VI Name"=w1037) -> ("Application reference"=w1035:refnum<vi>, "Path name"=w1034:path, "Local Call?"=w1036:bool)  [unwired: 2 out]
            n546 = global read "Dynamic_call_global.ph.vi" "Take LDA PWA & An"() -> (w1039:refnum<vi>)
            n547 = case shown="False" w1036 {
              tunnel: w1039 -> [w1045 w1049]
              tunnel: [w1041 w1048] -> w1038
              tunnel: [w1044 w1047] -> w1040
              tunnel: w1037 -> [w1043 _]
              tunnel: w1035 -> [w1042 _]
              tunnel: w1034 -> [_ w1046]
              frame False {
                n548 = Open VI Reference(type specifier VI Refnum (for type only)=w1045, application reference (local)=w1042, vi path=w1043) -> (vi reference=w1041:refnum<vi>, error out=w1044:errorcluster)  [unwired: 1 in, 2 out]
              }
              frame True {
                n549 = Open VI Reference(type specifier VI Refnum (for type only)=w1049, vi path=w1046) -> (vi reference=w1048:refnum<vi>, error out=w1047:errorcluster)  [unwired: 1 in, 3 out]
              }
            }
            n550 = global write "Dynamic_call_global.ph.vi" "Take LDA PWA & An"(w1038) -> ()
          }
          frame "Open vi" {
            n551 = local read "VI Name"() -> (w1054:string)
            n552 = call "Get_link_info.vi"("VI Name"=w1054) -> ("Application reference"=w1052:refnum<vi>, "Path name"=w1053:path, "Local Call?"=w1051:bool)  [unwired: 2 out]
            n553 = case shown="\"GPIB_Server.vi\"" w1054 {
              selector: w1054 -> [w1056 w1062 w1077]
              tunnel: [w1057 w1065 w1078] -> w1055
              tunnel: w1053 -> [_ _ w1079]
              tunnel: w1052 -> [_ w1064 w1081]
              tunnel: w1051 -> [_ w1063 w1080]
              frame "No Match", Default {
                n554 = Format Into String(format string="VI named \"%s\" Not matched" ("Format String"), w1056) -> (resulting string=w1059:string)  [unwired: 2 in, 1 out]
                n555 = Bundle By Name(cluster=errorcluster {"status"=FALSE, "code"=0, "source"=""} ("error out"), "source"=w1059, "status"=TRUE ("Bundle Element")) -> (w1057:errorcluster)
              }
              frame "Program_Active_server.vi" {
                n556 = global read "Dynamic_call_global.ph.vi" "Program Active server"() -> (w1067:refnum<vi>)
                n557 = case shown="True" w1063 {
                  tunnel: w1067 -> [w1072 w1076]
                  tunnel: [w1071 w1075] -> w1066
                  tunnel: [w1070 w1074] -> w1065
                  tunnel: w1062 -> [w1069 w1073]
                  tunnel: w1064 -> [w1068 _]
                  frame False {
                    n558 = Open VI Reference(type specifier VI Refnum (for type only)=w1072, application reference (local)=w1068, vi path=w1069) -> (vi reference=w1071:refnum<vi>, error out=w1070:errorcluster)  [unwired: 1 in, 2 out]
                  }
                  frame True {
                    n559 = Open VI Reference(type specifier VI Refnum (for type only)=w1076, vi path=w1073) -> (vi reference=w1075:refnum<vi>, error out=w1074:errorcluster)  [unwired: 1 in, 3 out]
                  }
                }
                n560 = global write "Dynamic_call_global.ph.vi" "Program Active server"(w1066) -> ()
              }
              frame "GPIB_Server.vi" {
                n561 = global read "Dynamic_call_global.ph.vi" "GPIB_Server.vi"() -> (w1083:refnum<vi>)
                n562 = case shown="False" w1080 {
                  tunnel: w1083 -> [w1088 w1092]
                  tunnel: [w1087 w1091] -> w1082
                  tunnel: [w1086 w1090] -> w1078
                  tunnel: w1077 -> [w1084 _]
                  tunnel: w1081 -> [w1085 _]
                  tunnel: w1079 -> [_ w1089]
                  frame False {
                    n563 = Open VI Reference(type specifier VI Refnum (for type only)=w1088, application reference (local)=w1085, vi path=w1084) -> (vi reference=w1087:refnum<vi>, error out=w1086:errorcluster)  [unwired: 1 in, 2 out]
                  }
                  frame True {
                    n564 = Open VI Reference(type specifier VI Refnum (for type only)=w1092, vi path=w1089) -> (vi reference=w1091:refnum<vi>, error out=w1090:errorcluster)  [unwired: 1 in, 3 out]
                  }
                }
                n565 = global write "Dynamic_call_global.ph.vi" "GPIB_Server.vi"(w1082) -> ()
              }
            }
          }
          frame "Update opened vis array" {
            w1097 = TRUE  # Dialog Box
            n566 = local read "VI Name"() -> (w1096:string)
            n567 = Unbundle By Name(w1095) -> ("status"=w1100:bool, "source"=w1098:string)
            n568 = case shown="True" w1100 {
              tunnel: w1095 -> [w1102 w1111]
              tunnel: [w1102 w1110] -> w1099
              tunnel: w1096 -> [w1103 w1106]
              tunnel: w1098 -> [_ w1109]
              frame False {
                n569 = To Upper Case(1:w1103) -> (0:w1101:string)
                n570 = global read "Dynamic_call_global.ph.vi" "Opened VIs"() -> (w1104:string[])
                n571 = Build Array (concatenate)(w1104, w1101) -> (w1105:string[])
                n572 = global write "Dynamic_call_global.ph.vi" "Opened VIs"(w1105) -> ()
              }
              frame True {
                n573 = Concatenate Strings(w1106, " " ("Substring"), w1109) -> (w1107:string)
                n574 = Bundle By Name(cluster=w1111, "source"=w1107) -> (w1110:errorcluster)
              }
            }
            n575 = call "EnFlo_Error_Handler.vi"("error in (no error)"=w1099, "Error Type"="Dynamic Call", "Dialog Box (F)"=w1097) -> ()  [unwired: 3 out]
          }
          frame "Wait until remote sub vi is opened" {
            n576 = global read "Dynamic_call_global.ph.vi" "Remote Subvi Opened"() -> (w1116:refnum<k4>)
            n577 = local read "Iterations"() -> (w1114:i32)
            n578 = Increment(x=w1114) -> (x+1=w1113:i32)
            n579 = local write "Iterations"(w1113) -> ()
            n580 = Set Occurrence(w1116) -> ()
          }
        }
      }
      n581 = disable-structure shown="TARGET_TYPE==Windows" {
        frame condition #0 (active) {
          n582 = while {
            stop <- FALSE stop-if-true
            n583 = stacked-sequence {
              frame #0 {
                n584 = global read "LDA_global.vi" "Connect BSA"() -> (w99:refnum<k4>)
                n585 = Wait on Occurrence(2:w99) -> ()  [unwired: 3 out]
              }
              frame #1 {
                n586 = global read "LDA_global.vi" "BSA IP Number"() -> (w104:string)
                n587 = global read "LDA_global.vi" "Connected BSA References"() -> (w103:refnum<k7>[])
                n588 = Automation Open(Automation Refnum=refnum<k7> refnum ("BSACtrl.IBSA 2"), 9:FALSE ("open new instance (false)")) -> (Automation Refnum=w108:refnum<k7>, error out=w109:errorcluster)  [unwired: 2 in]
                n589 = global read "LDA_global.vi" "Connected BSA IPs"() -> (w100:string[])
                n590 = invoke class="IBSA" method="Connect"(reference=w108, error in=w109, "ipaddress"=w104, "silent"=0) -> (reference out=w106:refnum<k7>, error out=w105:errorcluster)  [unwired: 1 in, 3 out]
                n591 = global write "LDA_global.vi" "Connect error out"(w105) -> ()
                n592 = case shown="No Error" w105 {
                  tunnel: w106 -> [w117 _]
                  tunnel: w104 -> [w116 w122]
                  tunnel: w103 -> [w115 w118]
                  tunnel: [w114 w119] -> w102
                  tunnel: [w113 w120] -> w101
                  tunnel: w100 -> [w112 w121]
                  frame No Error {
                    n593 = Build Array (concatenate)(w112, w116) -> (w113:string[])
                    n594 = Build Array (concatenate)(w115, w117) -> (w114:refnum<k7>[])
                  }
                  frame Error {
                    n595 = for {
                      tunnel: w122 -> [w126]
                      tunnel: w121 -> [w125] mode=indexing
                      tunnel: [w125] -> w120 mode=indexing if=w123
                      tunnel: [w124] -> w119 mode=indexing if=w123
                      tunnel: w118 -> [w124] mode=indexing
                      n596 = Not Equal?(x=w126, y=w125) -> (x != y?=w123:bool)
                    }
                  }
                }
                n597 = global write "LDA_global.vi" "Connected BSA IPs"(w101) -> ()
                n598 = global write "LDA_global.vi" "Connected BSA References"(w102) -> ()
              }
              frame #2 {
                n599 = global read "LDA_global.vi" "Connect BSA"() -> (w127:refnum<k4>)
                n600 = Set Occurrence(w127) -> ()
              }
            }
          }
          n601 = while {
            stop <- FALSE stop-if-true
            n602 = stacked-sequence {
              frame #0 {
                n603 = global read "LDA_global.vi" "Connect Laser Dx"() -> (w96:refnum<k4>)
                n604 = Wait on Occurrence(2:w96) -> ()  [unwired: 3 out]
              }
              frame #1 {
                n605 = call "Hub_Connect to Laser_Dx.vi"() -> ()  [unwired: 1 in]
              }
              frame #2 {
                n606 = global read "LDA_global.vi" "Connect Laser Dx"() -> (w97:refnum<k4>)
                n607 = Set Occurrence(w97) -> ()
              }
            }
          }
        }
        frame condition #1 {
        }
      }
      n608 = call "Last_modified_date.vi"("Update Now"=TRUE) -> ("concatenatedRevisions"=w88:string)  [unwired: 1 out]
      "Revision Info" <- w88
      n609 = while {
        i -> [w128]
        stop <- FALSE stop-if-true
        n610 = stacked-sequence {
          tunnel: w128 -> [w133 _ w204 w294]
          frame #0 {
            n611 = Quotient & Remainder(x=w133, y=3600) -> (x-y*floor(x/y)=w131:i32)  [unwired: 1 out]
            n612 = case shown="0" w131 {
              frame 0 {
                w134 = "LabVIEW:Administrators:"
                n613 = call "Get_Current_Scan_client.vi"("singleChannel"=w134) -> ("Ch Description Array"=w145:T42[])  [unwired: 1 in, 3 out]
                n614 = global read "Preference_global.vi" "Server Comms"() -> (w139:T41)
                n615 = Index Array(array=w145) -> (element=w144:T42)  [unwired: 1 in]
                n616 = Unbundle By Name(w144) -> ("String"=w143:string, "Ch Name"=w140:string)
                n617 = Equal?(x=Server_Comms."Do Not Link To Server" ("Server Comms"), y=w139) -> (x = y?=w136:bool)
                n618 = Equal?(x=w140, y="No:Match:") -> (x = y?=w135:bool)
                n619 = And(x=w135, y=w136) -> (x .and. y?=w137:bool)
                n620 = case shown="True" w137 {
                  tunnel: T42 {"Ch Name"="LabVIEW:Administrators:", "Type"="Hold Value", "Function"=enum."Analogue Input", "Ch State"=enum."On", "Calibration type"="Raw", "A"=0.0, "B"=0.0, "C"=0.0, "D"=0.0, "Comments"="", "Address"={"Main"=0, "Ch."=0, "Sub"=0, "Port Name"=""}, "String"="", "Duty"=1} ("element") -> [_ w149]
                  tunnel: w134 -> [_ w147]
                  frame False {
                  }
                  frame True {
                    n621 = Bundle By Name(cluster=w149, "Ch Name"=w147) -> (w148:T42)
                    n622 = Build Array(w148) -> (w150:T42[])
                    n623 = call "Update_Ch_Discription_client.vi"("Channels to update In"=w150) -> ()  [unwired: 1 in]
                  }
                }
                n624 = call "Get_array_values_fr_String.vi"("String Value"=w143) -> ("String array"=w146:string[])  [unwired: 1 out]
                n625 = global write "Preference_global.vi" "LabVIEW Administrators"(w146) -> ()
              }
              frame 1, Default {
              }
            }
          }
          frame #1 {
            n626 = Equal?(x="Tab Control", y=T1."Adam Table" ("Tab Control")) -> (x = y?=w151:bool)
            n627 = case shown="True" w151 {
              frame True {
                n628 = global read "Preference_global.vi" "Rig Setup"() -> (w161:string)
                n629 = local read "List of ADAM channels to view"() -> (w163:string[])
                n630 = Array Size(array=w163) -> (size(s)=w162:i32)
                n631 = local read "List of ADAM control channels"() -> (w170:string[])
                n632 = Build Array (concatenate)(w170, w163) -> (w158:string[])
                n633 = case shown="\"A_Tunnel\"" w161 {
                  tunnel: w158 -> [w173 w175 w178 w181 w184]
                  tunnel: [w173 w174 w177 w180 w183] -> w160
                  frame Default {
                  }
                  frame "EnFlo_Tunnel" {
                    n634 = Build Array (concatenate)(w175, "EnFlo_Tunnel:Reference:Velocity") -> (w174:string[])
                  }
                  frame "Aero_Tunnel" {
                    n635 = Build Array (concatenate)(w178, "Aero_Tunnel:Motor:Engaged") -> (w177:string[])
                  }
                  frame "A_Tunnel" {
                    n636 = Build Array (concatenate)(w181, "A_Tunnel:Speed:Meas Velocity") -> (w180:string[])
                  }
                  frame "D_Tunnel" {
                    n637 = Build Array (concatenate)(w184, "D_Tunnel:Speed:Meas Velocity") -> (w183:string[])
                  }
                }
                n638 = call "Get_Current_Scan_client.vi"("multipleChannels"=w160) -> ("Ch Description Array"=w167:T42[], "Numerical Values"=w159:dbl[])  [unwired: 1 in, 2 out]
                n639 = Array Size(array=w170) -> (size(s)=w168:i32)
                n640 = Array Subset(array=w167, index=w168, length=w162) -> (w166:T42[])
                n641 = Array Subset(array=w159, index=w168, length=w162) -> (w165:dbl[])
                n642 = for {
                  tunnel: w166 -> [w190] mode=indexing
                  tunnel: [w189] -> w164 mode=indexing
                  tunnel: cluster{"Ch Name":string, "Numeric":dbl} {"Ch Name"="", "Numeric"=0.0} ("Cluster") -> [w188]
                  tunnel: w165 -> [w186] mode=indexing
                  n643 = Unbundle By Name(w190) -> ("Ch Name"=w187:string)
                  n644 = Bundle By Name(cluster=w188, "Ch Name"=w187, "Numeric"=w186) -> (w189:cluster{"Ch Name":string, "Numeric":dbl})
                }
                "Current Values" <- w164
                n645 = for {
                  N: w168 -> [_]
                  tunnel: cluster{"Ch Name":string, "Boolean":bool} {"Ch Name"="", "Boolean"=FALSE} ("Cluster") -> [w203]
                  tunnel: w167 -> [w202] mode=indexing
                  tunnel: w159 -> [w200] mode=indexing
                  tunnel: [w197] -> w171 mode=indexing if=w191
                  n646 = Unbundle By Name(w202) -> ("Ch State"=w195:T45, "Ch Name"=w201:string)
                  n647 = Greater?(x=w200, y=0.5) -> (0:w198:bool)
                  n648 = Equal?(x=Channel_State."On" ("Ch State"), y=w195) -> (x = y?=w192:bool)
                  n649 = Equal?(x=Channel_State."Always On" ("Ch State"), y=w195) -> (x = y?=w193:bool)
                  n650 = Bundle By Name(cluster=w203, "Ch Name"=w201, "Boolean"=w198) -> (w197:cluster{"Ch Name":string, "Boolean":bool})
                  n651 = Or(x=w192, y=w193) -> (x .or. y?=w191:bool)
                }
                n652 = Array Size(array=w158) -> (size(s)=w157:i32)
                n653 = local write "Rig_Control"(w171) -> ()
                n654 = Index Array(array=w159, index=w157) -> (element=w156:dbl)
                n655 = Greater?(x=w156, y=0.15) -> (0:→"Tunnel Running?":bool)
              }
              frame False {
              }
            }
          }
          frame #2 {
            n656 = while {
              shift-right: [w209] -> _
              shift-left: "Start" -> [w211]
              tunnel: w204 -> [w208]
              shift-right: [w207] -> _
              shift-left: _ -> [w206]
              stop <- w210 continue-if-true
              n657 = case shown="\"Run monitor\"" w211 {
                selector: w211 -> [w212 _ _ _ _ _]
                tunnel: [FALSE TRUE TRUE TRUE FALSE FALSE] -> w210
                tunnel: ["End" "Check loopcount" w225 w232 "End" "End"] -> w209
                tunnel: w208 -> [_ _ w223 _ _ _]
                tunnel: [w213 w217 w219 w231 w262 w290] -> w207
                tunnel: w206 -> [w213 w217 w219 w231 w241 w290]
                frame "No Match", Default {
                  n658 = call "Case not matched.vi"("Case Name not Matched"=w212) -> ()
                }
                frame "Start" {
                }
                frame "Check loopcount" {
                  # "Only update every 10 cycles, which, based on 1000ms delay of outer loop equates to 10s sampling period"
                  # "(i MOD 10 == 0) reformulated to exclude first zero"
                  n659 = Quotient & Remainder(x=w223, y=11) -> (x-y*floor(x/y)=w221:i32)  [unwired: 1 out]
                  n660 = Equal?(x=w221, y=10) -> (x = y?=w220:bool)
                  n661 = Select(t="Check rig setup", s=w220, f="End") -> (s? t:f=w225:string)
                }
                frame "Check rig setup" {
                  n662 = global read "Coherent global.vi" "Number of connected devices"() -> (w230:u32)
                  n663 = Greater Than 0?(x=w230) -> (x > 0?=w229:bool)
                  n664 = Select(t="Run monitor", s=w229, f="End") -> (s? t:f=w232:string)
                }
                frame "Run monitor" {
                  w236 = errorcluster {"status"=FALSE, "code"=0, "source"=""} ("error in (no error)")
                  w259 = TRUE  # Don't Bother with check?
                  # "Call by reference to prevent loading of sub-hierarchy for rigs not using LDA. Treating the reference opening in this manner means it only ever has to be done once, and only if all checks are passed."
                  n665 = call-by-ref "Start Asynchronous Call"(reference=w241, error in=w236) -> (error out=w242:errorcluster)  [unwired: 2 in, 5 out]
                  n666 = call-by-ref "Wait On Asynchronous Call"(reference=w241, error in=w236) -> (reference out=w239:refnum<vi>, error out=w243:errorcluster, "GREEN LASER"=w238:T61, "BLUE LASER"=w237:T61)  [unwired: 2 in, 2 out]
                  n667 = Merge Errors(w242, w243) -> (w240:errorcluster)
                  n668 = case shown="Error" w240 {
                    selector: w240 -> [w273 _]
                    tunnel: [w274 w278] -> w262
                    tunnel: w239 -> [w274 _]
                    tunnel: [w273 w277] -> _
                    tunnel: [w272 w275] -> w261
                    tunnel: [w271 w276] -> w260
                    tunnel: w238 -> [w272 _]
                    tunnel: w237 -> [w271 _]
                    frame No Error {
                    }
                    frame Error {
                      n669 = Current VI's Path() -> (path=w287:path)
                      n670 = Strip Path(path=w287) -> (stripped path=w288:path)  [unwired: 1 out]
                      n671 = Build Path(base path=w288, name or relative path=path "Anemometry Sub Vis/LDA/Coherent/Lasers monitor ONESHOT.vi") -> (appended path=w285:path)
                      n672 = Open VI Reference(type specifier VI Refnum (for type only)=refnum<vi> refnum, vi path=w285, options=256, error in (no error)=errorcluster {"status"=FALSE, "code"=0, "source"=""}) -> (vi reference=w280:refnum<vi>, error out=w281:errorcluster)  [unwired: 2 in]
                      n673 = call-by-ref "Start Asynchronous Call"(reference=w280, error in=w281) -> (error out=w282:errorcluster)  [unwired: 2 in, 5 out]
                      n674 = call-by-ref "Wait On Asynchronous Call"(reference=w280, error in=w281) -> (reference out=w278:refnum<vi>, error out=w279:errorcluster, "GREEN LASER"=w275:T61, "BLUE LASER"=w276:T61)  [unwired: 2 in, 2 out]
                      n675 = Merge Errors(w282, w279) -> (w277:errorcluster)
                    }
                  }
                  n676 = Unbundle By Name(w261) -> ("Power (mW)"=w258:sgl, "LDD current (A)"=w257:sgl, "TEC drive (V)"=w256:sgl, "TEC temp. (degC)"=w255:sgl, "SHG heater (degC)"=w254:sgl, "BRF heater (degC)"=w253:sgl)
                  n677 = Unbundle By Name(w260) -> ("Power (mW)"=w252:sgl, "LDD current (A)"=w251:sgl, "TEC drive (V)"=w250:sgl, "TEC temp. (degC)"=w249:sgl, "SHG heater (degC)"=w248:sgl, "BRF heater (degC)"=w247:sgl)
                  n678 = Build Array(w258, w257, w256, w255, w254, w253, w252, w251, w250, w249, w248, w247) -> (w246:sgl[])
                  n679 = for {
                    tunnel: string[] ["LDA1:Green:Power (mW)", "LDA1:Green:LDD current (A)", "LDA1:Green:TEC drive (V)", "LDA1:Green:TEC temp. (degC)", "LDA1:Green:SHG heater (degC)", "LDA1:Green:BRF heater (degC)", "LDA1:Blue:Power (mW)", "LDA1:Blue:LDD current (A)", "LDA1:Blue:TEC drive (V)", "LDA1:Blue:TEC temp. (degC)", "LDA1:Blue:SHG heater (degC)", "LDA1:Blue:BRF heater (degC)"] -> [w269] mode=indexing
                    tunnel: w246 -> [w268] mode=indexing
                    tunnel: [w266] -> w245 mode=indexing
                    n680 = To Double Precision Float(number=w268) -> (double precision float=w267:dbl)
                    n681 = Bundle By Name(cluster=T48 {"Channel Name"="", "New Value"=0.0, "!Auto_Off"=FALSE} ("Update Scan Value Cluster"), "Channel Name"=w269, "New Value"=w267, "!Auto_Off"=TRUE) -> (w266:T48)
                  }
                  n682 = call "Update_Current_Value_client.vi"("Don't Bother with check?"=w259, "Update array in"=w245) -> ()
                }
                frame "End" {
                }
              }
            }
          }
          frame #3 {
            n683 = global read "LDA_global.vi" "Connected Laser Dx Refs"() -> (w293:refnum<k7>[])
            n684 = while {
              shift-right: [w298] -> _
              shift-left: "Start" -> [w300]
              tunnel: w294 -> [w297]
              tunnel: w293 -> [w296]
              stop <- w299 continue-if-true
              n685 = case shown="\"Log Dx Lasers\"" w300 {
                selector: w300 -> [w303 _ _ _ _]
                tunnel: [FALSE TRUE TRUE TRUE FALSE] -> w299
                tunnel: ["End" "Check loopcount" w320 "End" "End"] -> w298
                tunnel: w297 -> [_ _ w318 _ _]
                tunnel: w296 -> [_ _ w315 w331 _]
                frame "No Match", Default {
                  n686 = Current VI's Path() -> (path=w308:path)
                  n687 = Format Into String(format string="The Case\"%s\" was not Matched\nin VI named\n'%s\"" ("Format String"), w303, w308) -> (resulting string=w305:string)  [unwired: 2 in, 1 out]
                  n688 = One Button Dialog(message=w305, button name ("OK")="STOP") -> (true=w307:bool)
                  n689 = Stop(stop? (T)=w307) -> ()
                }
                frame "Start" {
                }
                frame "Check loopcount" {
                  # "Only update every 30 cycles, which, based on 1000ms delay of outer loop equates to 30s sampling period"
                  # "(i MOD 10 == 0) reformulated to exclude first zero"
                  n690 = Array Size(array=w315) -> (size(s)=w314:i32)
                  n691 = Greater Than 0?(x=w314) -> (x > 0?=w312:bool)
                  n692 = Quotient & Remainder(x=w318, y=31) -> (x-y*floor(x/y)=w316:i32)  [unwired: 1 out]
                  n693 = Equal?(x=w316, y=10) -> (x = y?=w313:bool)
                  n694 = And(x=w312, y=w313) -> (x .and. y?=w311:bool)
                  n695 = Select(t="Log Dx Lasers", s=w311, f="End") -> (s? t:f=w320:string)
                }
                frame "Log Dx Lasers" {
                  n696 = global read "LDA_global.vi" "Connected Laser Dx number"() -> (w330:i64[])
                  n697 = global read "LDA_global.vi" "Available Laser Dx names"() -> (w332:string[])
                  n698 = global read "LDA_global.vi" "Connected Laser Dx IPs"() -> (w326:string[])
                  n699 = for {
                    tunnel: w331 -> [w344] mode=indexing
                    tunnel: T48 {"Channel Name"="", "New Value"=0.0, "!Auto_Off"=TRUE} ("Update Scan Value Cluster") -> [w358]
                    tunnel: w332 -> [w337] mode=indexing
                    tunnel: w330 -> [w345] mode=indexing
                    tunnel: [w345] -> w329 mode=indexing if=w338
                    tunnel: [w344] -> w328 mode=indexing if=w338
                    tunnel: [w348] -> w327 mode=indexing if=w338
                    tunnel: w326 -> [w348] mode=indexing
                    tunnel: [w336] -> w324 mode=concatenating
                    w339 = nan
                    # "Meas Power"
                    # "Hours"
                    n700 = disable-structure shown="TARGET_TYPE!=Windows, Default" {
                      disable-tunnel: [w369 "" ("GetStatus")] -> w347
                      disable-tunnel: [w368 errorcluster {"status"=FALSE, "code"=0, "source"=""} ("error out")] -> w346
                      disable-tunnel: w345 -> [w367 _]
                      disable-tunnel: w344 -> [w366 _]
                      frame condition #0 (active) {
                        n701 = invoke class="IBSALaser" method="GetStatus"(reference=w366, "dev"=w367) -> (error out=w368:errorcluster, "GetStatus"=w369:string)  [unwired: 3 in, 3 out]
                      }
                      frame condition #1 {
                      }
                    }
                    n702 = while {
                      shift-right: [w380] -> _
                      shift-left: w347 -> [w382]
                      tunnel: [w377] -> w359 mode=indexing
                      stop <- w381 stop-if-true
                      n703 = Match Pattern(string=w382, regular expression=";") -> (before substring=w379:string, after substring=w380:string)  [unwired: 1 in, 2 out]
                      n704 = Empty String/Path?(string/path=w380) -> (empty?=w381:bool)
                      n705 = Match Pattern(string=w379, regular expression=":") -> (after substring=w377:string)  [unwired: 1 in, 3 out]
                    }
                    n706 = Index Array(array=w359, index #1=2 ("index"), index #2=3 ("index")) -> (element #1=w362:string, element #2=w363:string)
                    n707 = Unbundle By Name(w346) -> ("status"=w357:bool)
                    n708 = Fract/Exp String To Number(string=w363) -> (number=w341:dbl)  [unwired: 3 in, 1 out]
                    n709 = Fract/Exp String To Number(string=w362) -> (number=w343:dbl)  [unwired: 3 in, 1 out]
                    n710 = Equal To 0?(x=w341) -> (x = 0?=w356:bool)
                    n711 = Compound Arithmetic op=AND(w356, invert w357) -> (w355:bool)
                    n712 = Concatenate Strings(w337, ":Meas Power (mW)" ("string")) -> (w353:string)
                    n713 = Concatenate Strings(w337, ":Hours" ("string")) -> (w351:string)
                    n714 = case shown="True" w355 {
                      tunnel: [w372 w373] -> w350
                      tunnel: w346 -> [w372 w376]
                      tunnel: w351 -> [_ w374]
                      frame False {
                      }
                      frame True {
                        n715 = Bundle By Name(cluster=w376, "status"=TRUE, "source"=w374) -> (w373:errorcluster)
                      }
                    }
                    n716 = Unbundle By Name(w350) -> ("status"=w349:bool)
                    n717 = Not(x=w349) -> (.not. x?=w338:bool)
                    n718 = Select(t=w341, s=w338, f=w339) -> (s? t:f=w340:dbl)
                    n719 = Select(t=w343, s=w338, f=w339) -> (s? t:f=w342:dbl)
                    n720 = Bundle By Name(cluster=w358, "Channel Name"=w353, "New Value"=w342) -> (w364:T48)
                    n721 = Bundle By Name(cluster=w358, "Channel Name"=w351, "New Value"=w340) -> (w365:T48)
                    n722 = Build Array(w364, w365) -> (w336:T48[])
                  }
                  n723 = call "Update_Current_Value_client.vi"("Don't Bother with check?"=TRUE, "Update array in"=w324) -> ()
                  n724 = global write "LDA_global.vi" "Connected Laser Dx number"(w329) -> ()
                  n725 = global write "LDA_global.vi" "Connected Laser Dx IPs"(w327) -> ()
                  n726 = global write "LDA_global.vi" "Connected Laser Dx Refs"(w328) -> ()
                }
                frame "End" {
                }
              }
            }
          }
        }
        n727 = Wait (ms)(milliseconds to wait=u32 1000) -> ()  [unwired: 1 out]
      }
      n728 = global write "Meas_global.vi" "ProgRevisionInfo"(w88) -> ()
      n729 = while {
        stop <- FALSE stop-if-true
        n730 = Get Date/Time In Seconds() -> (seconds since 1Jan1904=w94:timestamp)
        n731 = To Double Precision Float(number=w94) -> (double precision float=w93:dbl)
        n732 = global write "Dynamic_call_global.ph.vi" "EnFlo Hub last spoke"(w93) -> ()
        n733 = Wait (ms)(milliseconds to wait=u32 300) -> ()  [unwired: 1 out]
      }
    }
  }
